vi "3D Experiment Final wii.vi"() -> ()   [LabVIEW 2011]
uses:
  <vilib>/Utility/miscctls.llb/LV3DPointTypeDef.ctl
  <vilib>/Platform/TimedLoop/XDataNode/timing_clust.ctl
  <vilib>/Platform/TimedLoop/XDataNode/nitl_modes.ctl
  <vilib>/Platform/TimedLoop/XDataNode/wakeup.ctl
  <vilib>/Utility/miscctls.llb/LVRGBAColorTypeDef.ctl
  <vilib>/Utility/cursorutil.llb/Set Cursor (Cursor ID).vi
  libs/experiments 2/Action Engines/AE Access VIs/AE - Bluetooth Initialise.vi
  libs/experiments 2/Action Engines/AE Access VIs/AE - Bluetooth Connect All.vi
  <vilib>/Utility/file.llb/Write To Spreadsheet File (DBL).vi
  <vilib>/Utility/file.llb/Write To Spreadsheet File (I64).vi
  <vilib>/Platform/TimedLoop/XDataNode/XDataNode.xnode
  <vilib>/picture/3D Picture Control/NI_3D Picture Control.lvlib
  User32.dll
  <vilib>/Platform/TimedLoop/XDataNode/XDNodeRunTimeDep.lvlib
panel:
  out "initial time 2":u32
  out "initial time":u32
  in  "stop":bool
  out "3D Picture":refnum<vi>(3d-picture)
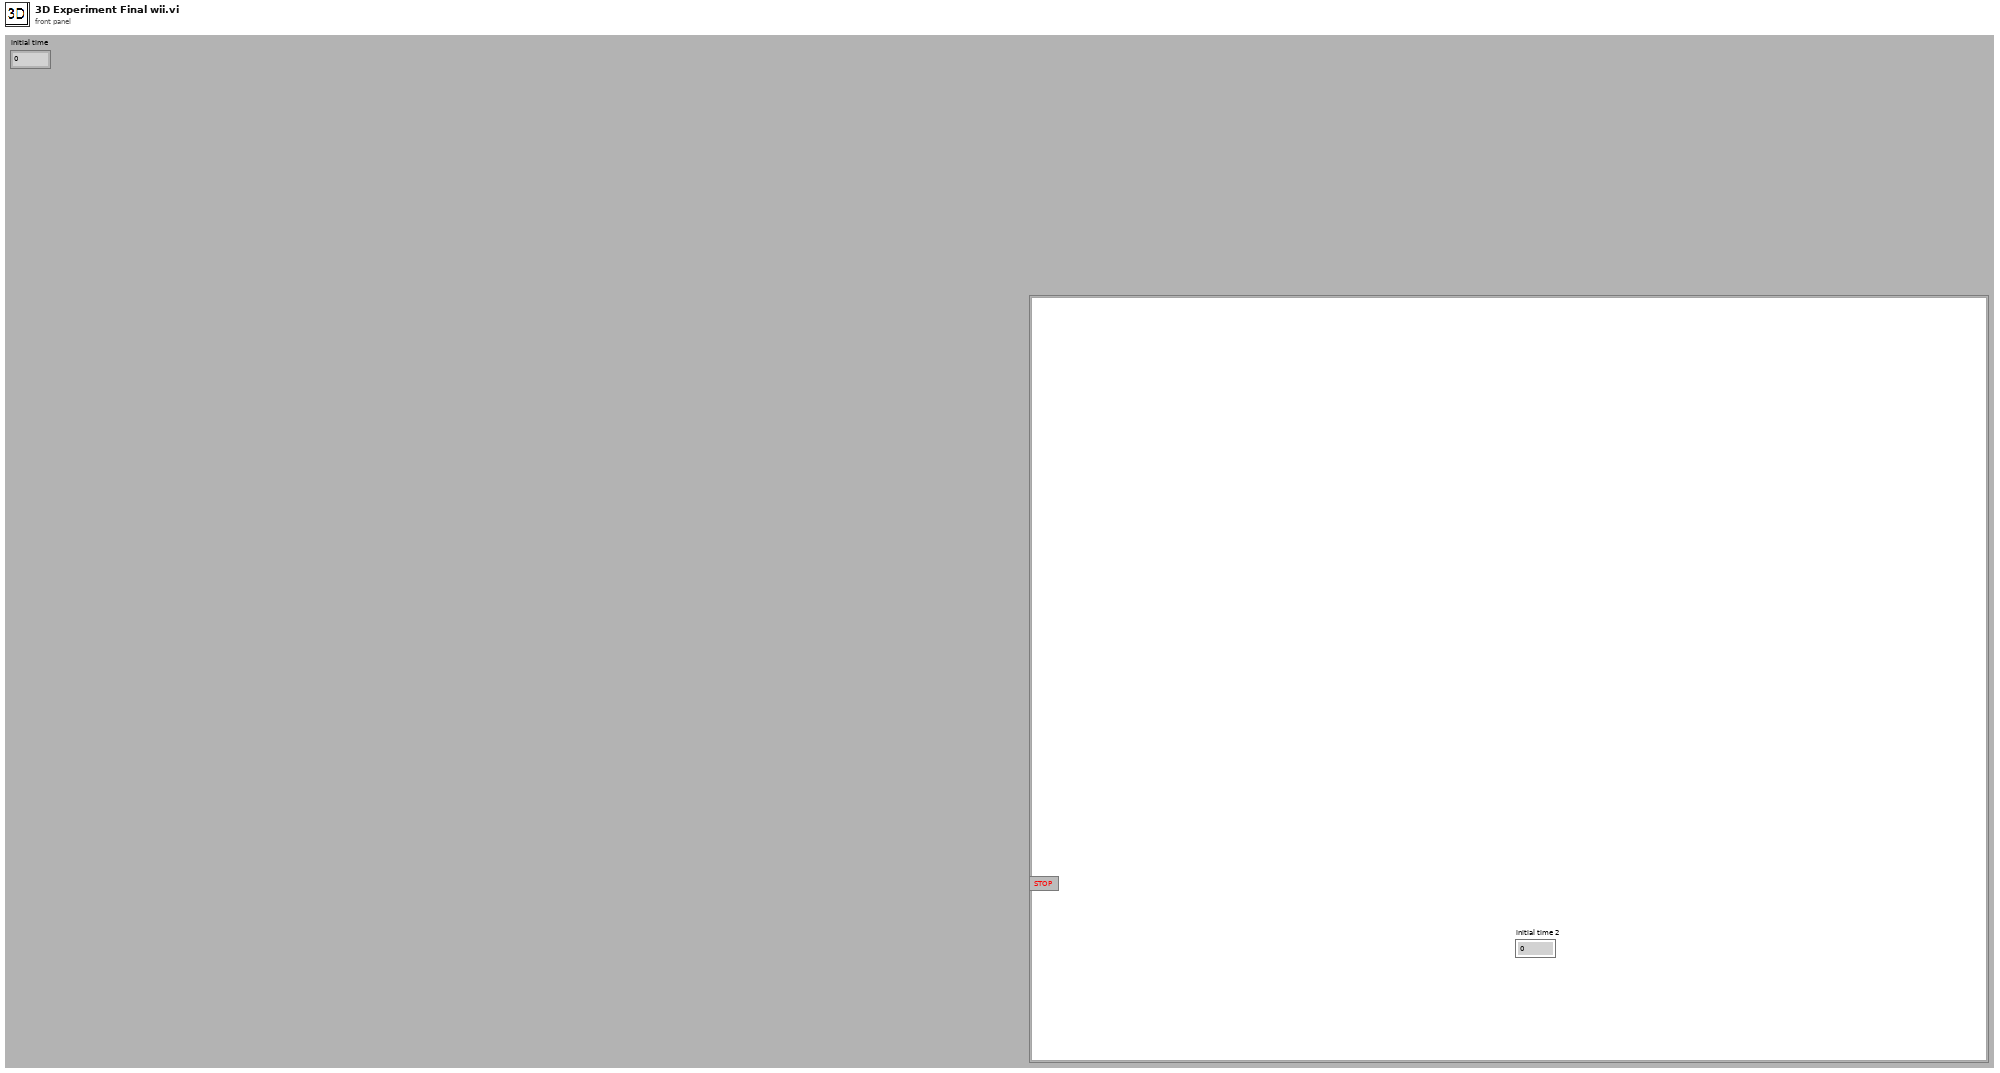
[diagram p1: front panel]
types:
  T1 = enum16{"open", "replace", "create", "open or create", "replace or create", "replace or create with confirmation"}
  T2 = typedef "LV3DPointTypeDef.ctl" = cluster{"X":sgl, "Y":sgl, "Z":sgl}
  T3 = enum16{"Inherit Value", "Points", "Wireframe", "Polygons"}
  T4 = enum16{"Inherit Value", "No Culling", "Cull Back Face", "Cull Front Face", "Cull Both Faces"}
  T5 = enum16{"Zero", "One", "Destination Color", "One Minus Destination Color", "Source Alpha", "One Minus Source Alpha", "Destination Alpha", "One Minus Destination Alpha", "Source Alpha Saturate"}
  T6 = enum16{"Zero", "One", "Source Color", "One Minus Source Color", "Source Alpha", "One Minus Source Alpha", "Destination Alpha", "One Minus Destination Alpha"}
  T7 = enum16{"Normal Bin", "Opaque Bin", "Transparent Bin"}
  T8 = typedef "XDNodeRunTimeDep.lvlib/timing_clust.ctl" = cluster{"Expected End [f-1]":u64, "Actual End [f-1]":u64, "Finished Late? [f-1]":bool, "Expected End [i-1]":u64, "Actual End [i-1]":u64, "Finished Late? [i-1]":bool, "Expected Start [i]":u64, "Actual Start [i]":u64, "Expected Start [f]":u64, "Actual Start [f]":u64, "Source Name":string, "Structure Name":string, "Period":i64, "Deadline":i64, "Offset":i64, "Start":i64, "Priority":i32, "Timeout":i32, "Mode":T9, "Wakeup Reason":T10, "Error":errorcluster, "Source Type":string, "Secondary Source Type":string, "Global End Time":u64, "Global Start Time":u64, "Frame Duration":u64, "Iteration Duration":u64, "Assigned CPU":i32, "I/O Scan Engine Mode":u32}
  T9 = typedef "XDNodeRunTimeDep.lvlib/nitl_modes.ctl" = enum32{"No Change", "Process missed periods, maintain original phase", "Discard missed periods, maintain original phase", "Process missed periods, ignore original phase", "Discard missed periods, ignore original phase"}
  T10 = typedef "XDNodeRunTimeDep.lvlib/wakeup.ctl" = enum32{"Normal", "Aborted", "Asynchronous wakeup", "Timing source error", "Timed loop error", "Timeout"}
  T11 = cluster{"Red":sgl, "Green":sgl, "Blue":sgl, "Alpha":sgl}
  T12 = typedef "LVRGBAColorTypeDef.ctl" = cluster{"Red":sgl, "Green":sgl, "Blue":sgl, "Alpha":sgl}
  T13 = typedef "LVAllMonitorsDisplayTypeDef.ctl" = cluster{"Bounds":cluster{"Left":i16, "Top":i16, "Right":i16, "Bottom":i16}, "Depth":i16}[]
  T14 = cluster{"Bounds":cluster{"Left":i16, "Top":i16, "Right":i16, "Bottom":i16}, "Depth":i16}
  T15 = cluster{"Left":i16, "Top":i16, "Right":i16, "Bottom":i16}
  T16 = cluster{"element":dbl, "Y_scaling":dbl, "element":dbl}
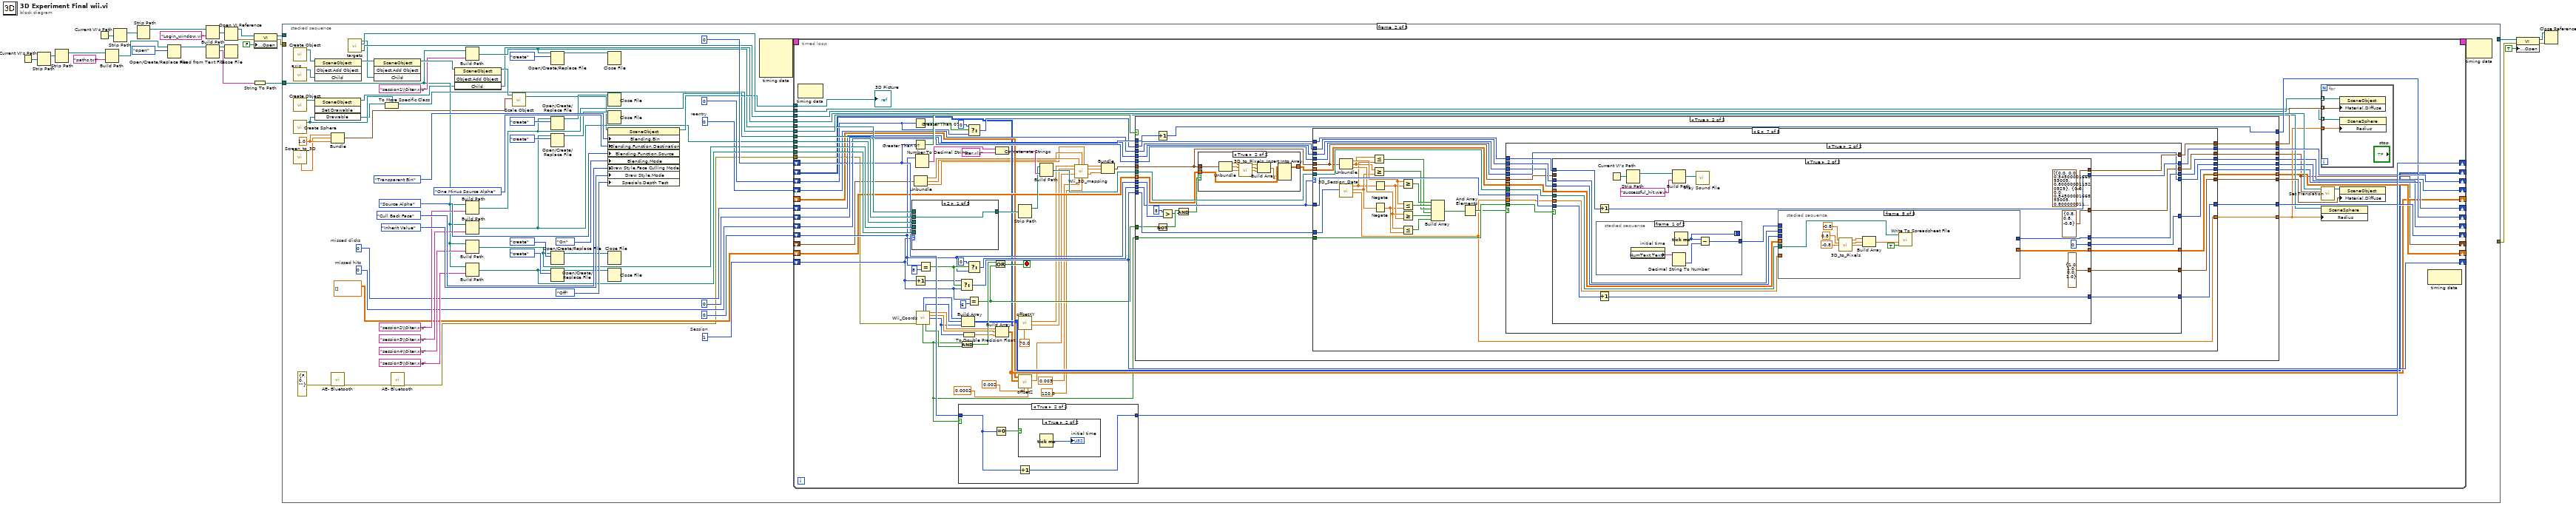
[diagram p0: block diagram]
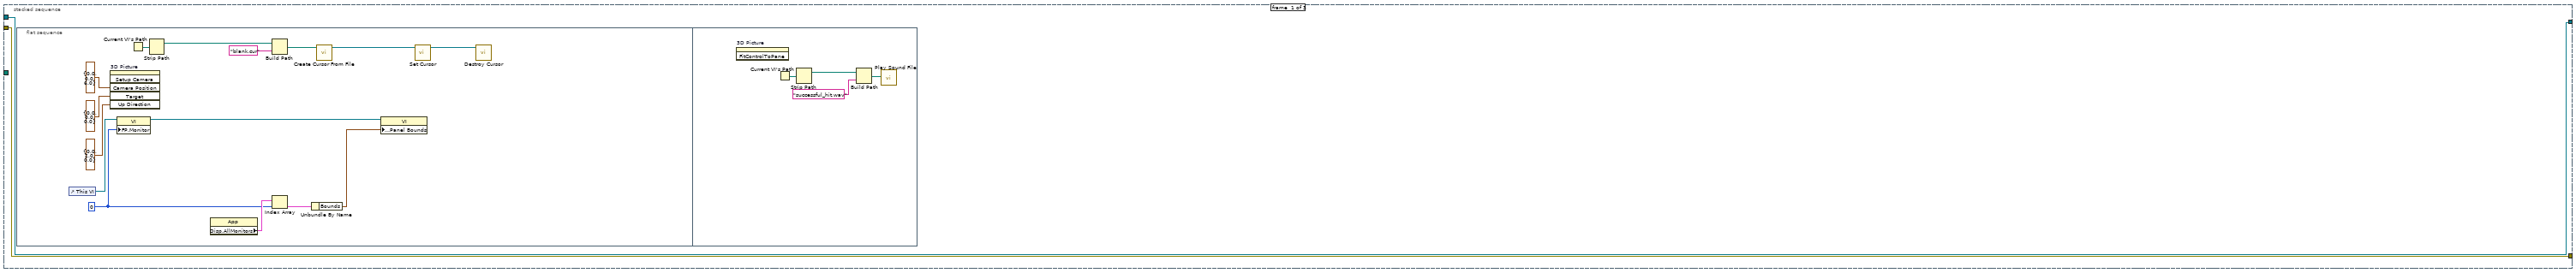
[diagram p2: hidden frame]
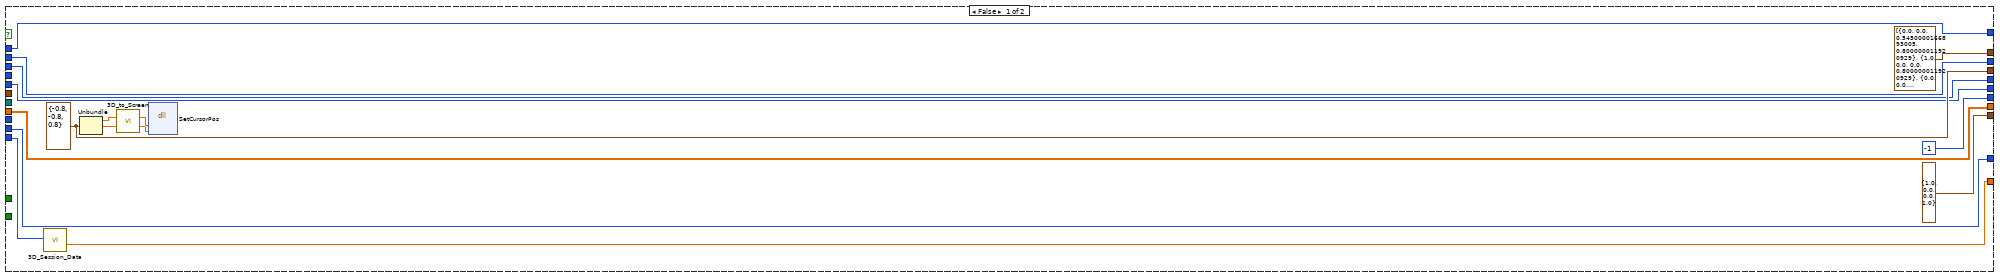
[diagram p7: hidden frame]
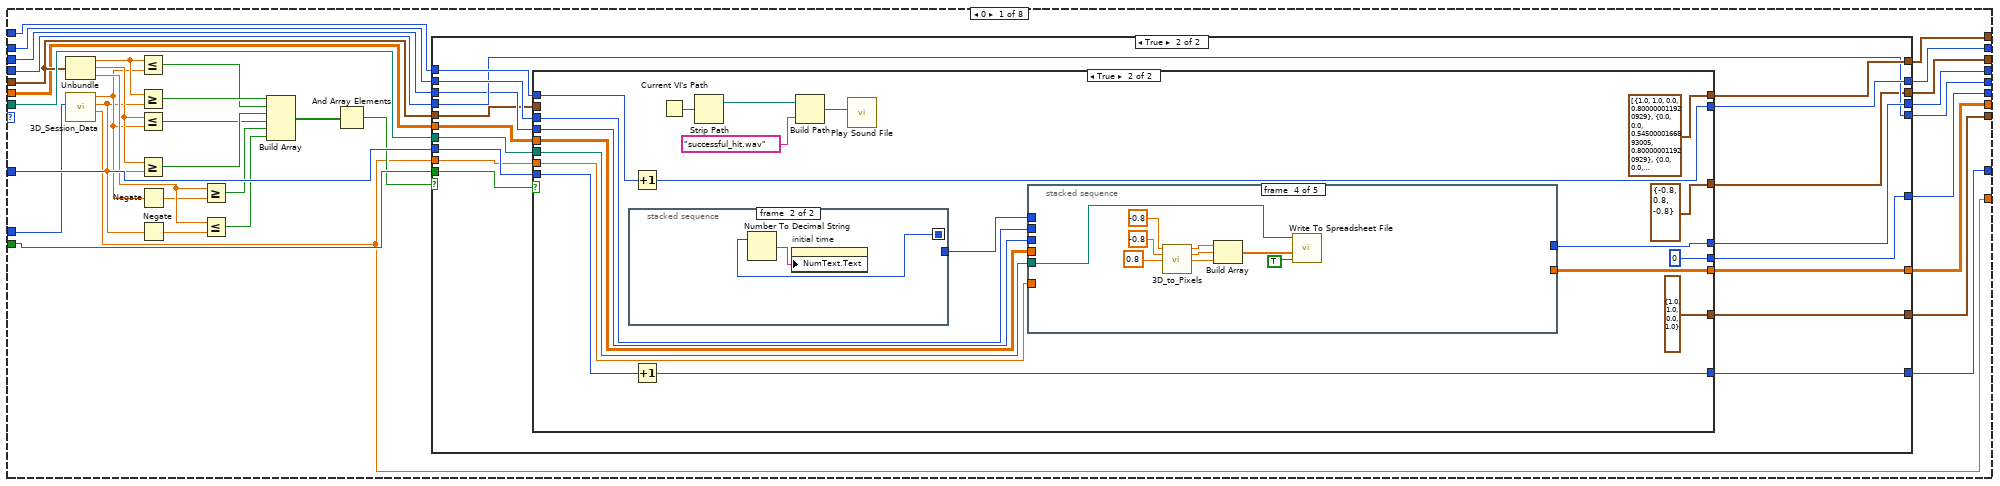
[diagram p9: hidden frame]
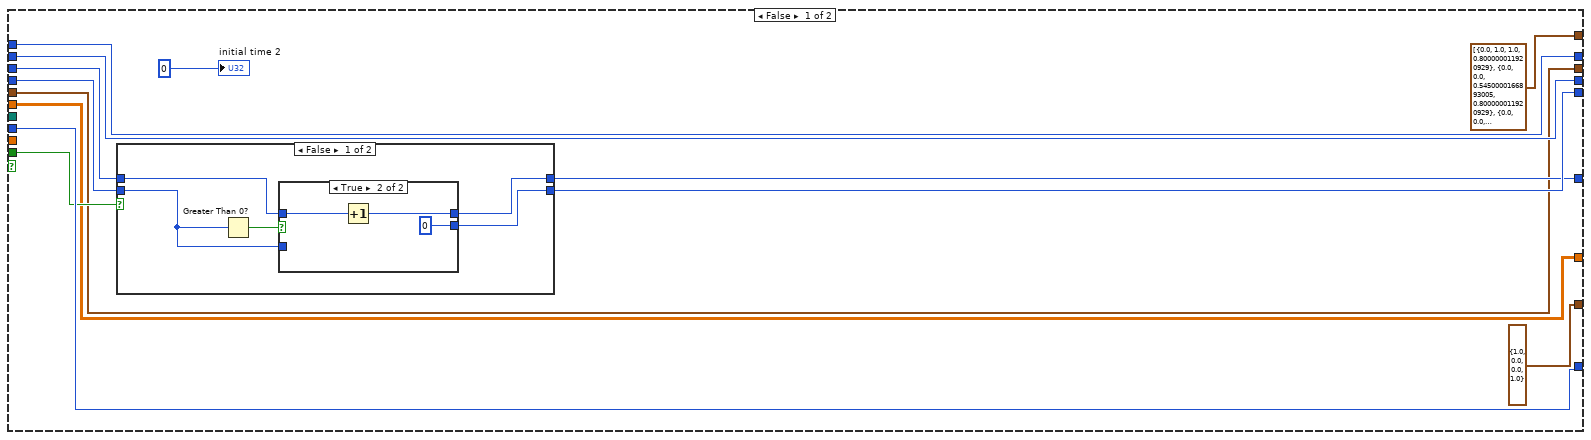
[diagram p10: hidden frame]
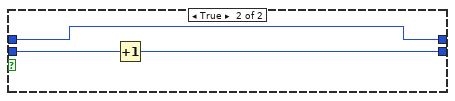
[diagram p12: hidden frame]
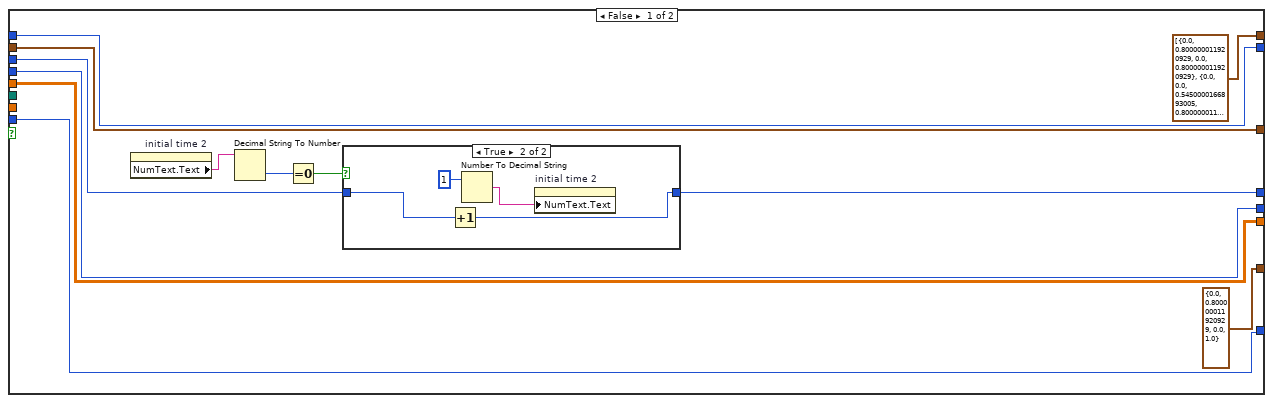
[diagram p13: hidden frame]
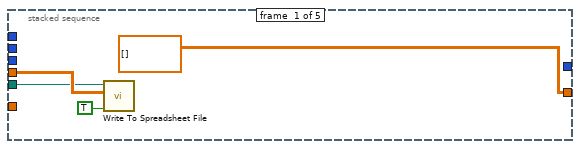
[diagram p15: hidden frame]
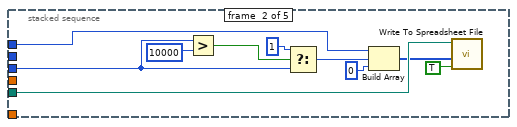
[diagram p16: hidden frame]
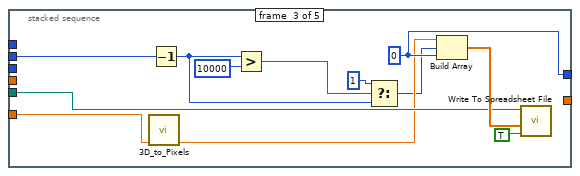
[diagram p17: hidden frame]
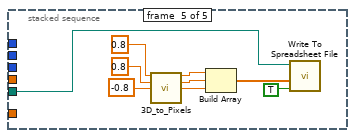
[diagram p18: hidden frame]
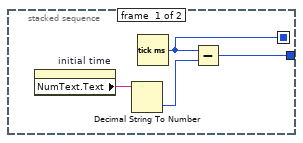
[diagram p19: hidden frame]
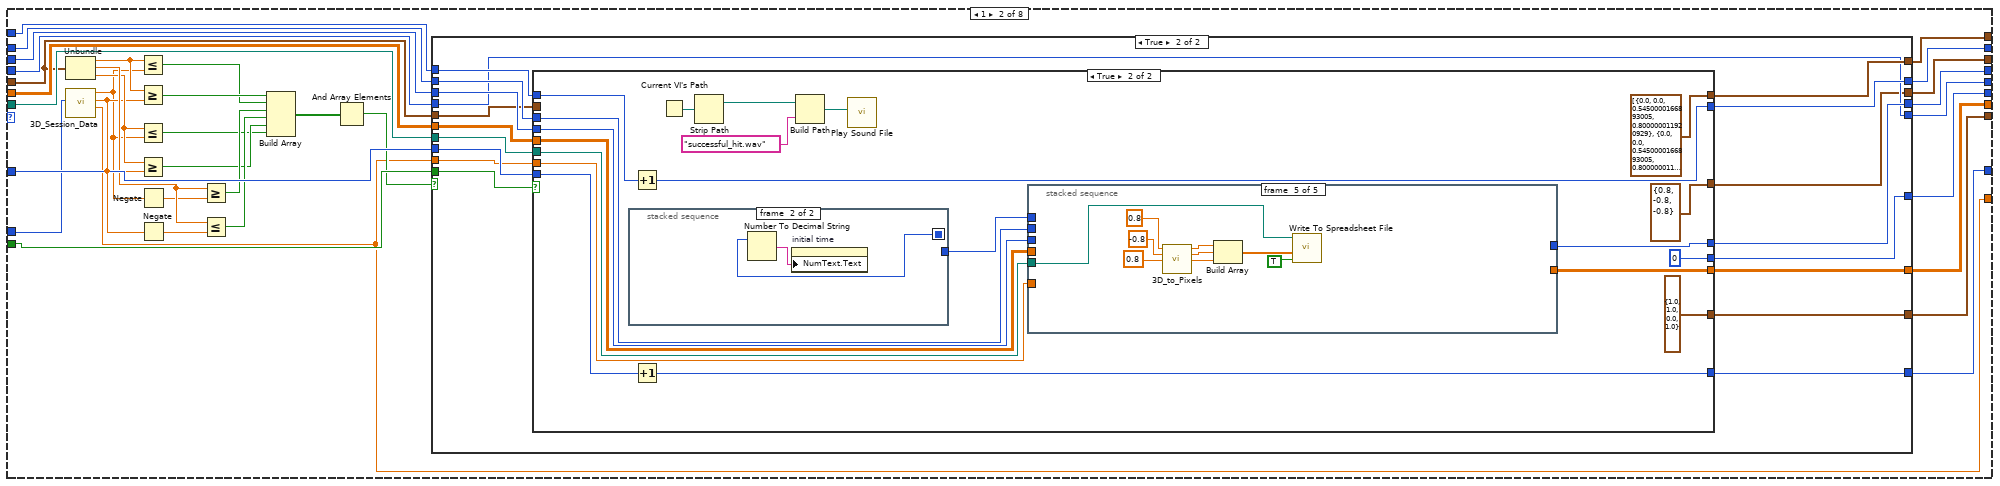
[diagram p20: hidden frame]
diagram:
  n1 = Current VI's Path() -> (path=w1:path)
  n2 = Strip Path(path=w1) -> (stripped path=w2:path)  [unwired: 1 out]
  n3 = Strip Path(path=w2) -> (stripped path=w19:path)  [unwired: 1 out]
  n4 = Current VI's Path() -> (path=w14:path)
  n5 = Build Path(base path=w19, name or relative path="paths.txt") -> (appended path=w22:path)
  n6 = Strip Path(path=w14) -> (stripped path=w11:path)  [unwired: 1 out]
  n7 = Strip Path(path=w11) -> (stripped path=w10:path)  [unwired: 1 out]
  n8 = Open/Create/Replace File(file path (use dialog)=w22, operation (0:open)=T1."open") -> (refnum out=w24:refnum<file>)  [unwired: 4 in, 2 out]
  n9 = Build Path(base path=w10, name or relative path="Login_window.vi") -> (appended path=w12:path)
  n10 = Read from Text File(file (use dialog)=w24) -> (refnum out=w25:refnum<file>, text=w23:string)  [unwired: 3 in, 2 out]
  n11 = Open VI Reference(vi path=w12) -> (vi reference=w17:refnum<vi>, error out=w16:errorcluster)  [unwired: 5 in]
  n12 = Close File(refnum=w25) -> ()  [unwired: 1 in, 2 out]
  n13 = String To Path(string=w23) -> (path=w18:path)
  n14 = property class="VI"(reference=w17, error in=w16, "Front Panel Window:Open"=FALSE) -> (reference out=w9:refnum<vi>, error out=w8:errorcluster)
  n15 = stacked-sequence {
    tunnel: w18 -> [_ w67 _]
    tunnel: w9 -> [w27 _ _]
    tunnel: w8 -> [w26 _ _]
    tunnel: [w27 _ _] -> w4
    tunnel: [w26 _ _] -> w3
    frame #0 {
      n16 = flat-sequence {
        frame #0 {
          w39 = u16 0 ("Front Panel Window:Monitor")
          n17 = control-ref of="This VI"() -> (w37:refnum<vi>)
          n18 = invoke on="3D Picture" class="SceneGraphDisp (strict)" method="Setup Camera"("Camera Position"=T2 {"X"=0.0, "Y"=0.0, "Z"=6.0}, "Target"=T2 {"X"=0.0, "Y"=0.0, "Z"=0.0}, "Up Direction"=T2 {"X"=0.0, "Y"=2.0, "Z"=0.0}) -> ()  [unwired: 3 in, 6 out]
          n19 = property class="VI"(reference=w37, "FP.Monitor"=w39) -> (reference out=w41:refnum<vi>)  [unwired: 1 in, 1 out]
          n20 = Current VI's Path() -> (path=w36:path)
          n21 = Strip Path(path=w36) -> (stripped path=w35:path)  [unwired: 1 out]
          n22 = property class="App"() -> ("Disp.AllMonitors"=w40:T13)  [unwired: 2 in, 2 out]
          n23 = Build Path(base path=w35, name or relative path="blank.cur") -> (appended path=w33:path)
          n24 = Index Array(array=w40, index=w39) -> (element=w38:T14)
          n25 = Unbundle By Name(w38) -> ("Bounds"=w42:T15)
          n26 = call <vilib>:"Create Cursor From File.vi"("cursor file"=w33) -> ("cursor ID"=w32:refnum<k1>)  [unwired: 9 in, 1 out]
          n27 = property class="VI"(reference=w41, "Front Panel Window:Panel Bounds"=w42) -> ()  [unwired: 1 in, 2 out]
          n28 = call-poly <vilib>:"Set Cursor.vi"("cursor ID"=w32) -> ("previous cursor ID"=w31:refnum<k1>)  [unwired: 9 in, 1 out]
          n29 = call <vilib>:"Destroy Cursor.vi"("cursor ID"=w31) -> ()  [unwired: 9 in, 1 out]
        }
        frame #1 {
          n30 = invoke on="3D Picture" class="SceneGraphDisp (strict)" method="FitControlToPane"() -> ()  [unwired: 3 in, 3 out]
          n31 = Current VI's Path() -> (path=w45:path)
          n32 = Strip Path(path=w45) -> (stripped path=w44:path)  [unwired: 1 out]
          n33 = Build Path(base path=w44, name or relative path="successful_hit.wav") -> (appended path=w46:path)
          n34 = call <vilib>:"Play Sound File.vi"("path"=w46) -> ()  [unwired: 9 in, 2 out]
        }
      }
    }
    frame #1 {
      w54 = 1.0 ("element")
      w55 = 0  # missed clicks
      w56 = 0  # missed hits
      w57 = 0  # reentry
      w96 = 1  # Session
      n35 = call <vilib>:"Create Object.vi"() -> ("Scene:New Object"=w100:refnum<vi>)  [unwired: 10 in, 1 out]
      n36 = call "axis.vi"() -> ("reference out"=w59:refnum<vi>)  [unwired: 11 in]
      n37 = call <vilib>:"Create Object.vi"() -> ("Scene:New Object"=w101:refnum<vi>)  [unwired: 10 in, 1 out]
      n38 = call <vilib>:"Create Sphere.vi"() -> ("New Sphere Refnum"=w94:refnum<vi>)  [unwired: 10 in, 1 out]
      n39 = call "Screen_to_3D.vi"() -> ("Y_scaling"=w51:dbl)  [unwired: 13 in, 6 out]
      n40 = invoke class="SceneObject" method="Object.Add Object"(reference=w100, "Child"=w59) -> (reference out=w99:refnum<vi>)  [unwired: 2 in, 3 out]
      n41 = invoke class="SceneObject" method="Set Drawable"(reference=w101, "Drawable"=w94) -> (reference out=w60:refnum<vi>, "Drawable"=w93:refnum<vi>)  [unwired: 2 in, 2 out]
      n42 = call-poly "AE- Bluetooth.vi"("error in (no error)"=errorcluster {"status"=FALSE, "code"=0, "source"=""}) -> ("error out"=w48:errorcluster)  [unwired: 10 in]
      n43 = Bundle("element"=w54, "Y_scaling"=w51, "element"=w54) -> (w53:T16)  [unwired: 1 in]
      n44 = call "targets.vi"() -> ("objects"=w95:refnum<vi>[], "shperes"=w91:refnum<vi>[], "Scene:New Object"=w58:refnum<vi>)  [unwired: 8 in]
      n45 = invoke class="SceneObject" method="Object.Add Object"(reference=w99, "Child"=w58) -> (reference out=w98:refnum<vi>)  [unwired: 2 in, 3 out]
      n46 = To More Specific Class(target class=w94, reference=w93) -> (specific class reference=w92:refnum<vi>)  [unwired: 1 in, 1 out]
      n47 = call-poly "AE- Bluetooth.vi"("error in (no error)"=w48) -> ("error out"=w47:errorcluster)  [unwired: 9 in, 1 out]
      n48 = invoke class="SceneObject" method="Object.Add Object"(reference=w98, "Child"=w60) -> (reference out=w97:refnum<vi>, "Child"=w61:refnum<vi>)  [unwired: 2 in, 2 out]
      n49 = Build Path(base path=w67, name or relative path="session1\\0iter.xls") -> (appended path=w62:path)
      n50 = Build Path(base path=w67, name or relative path="session2\\0iter.xls") -> (appended path=w63:path)
      n51 = Build Path(base path=w67, name or relative path="session3\\0iter.xls") -> (appended path=w65:path)
      n52 = Build Path(base path=w67, name or relative path="session4\\0iter.xls") -> (appended path=w64:path)
      n53 = Build Path(base path=w67, name or relative path="session5\\0iter.xls") -> (appended path=w66:path)
      n54 = call <vilib>:"Scale Object.vi"("Scale"=w53, "Scene.Object In"=w97) -> ("Scene.Object Out"=w52:refnum<vi>)  [unwired: 8 in, 1 out]
      n55 = Open/Create/Replace File(file path (use dialog)=w62, operation (0:open)=T1."create") -> (refnum out=w75:refnum<file>)  [unwired: 4 in, 2 out]
      n56 = Open/Create/Replace File(file path (use dialog)=w63, operation (0:open)=T1."create") -> (refnum out=w77:refnum<file>)  [unwired: 4 in, 2 out]
      n57 = Open/Create/Replace File(file path (use dialog)=w65, operation (0:open)=T1."create") -> (refnum out=w72:refnum<file>)  [unwired: 4 in, 2 out]
      n58 = Open/Create/Replace File(file path (use dialog)=w64, operation (0:open)=T1."create") -> (refnum out=w69:refnum<file>)  [unwired: 4 in, 2 out]
      n59 = Open/Create/Replace File(file path (use dialog)=w66, operation (0:open)=T1."create") -> (refnum out=w70:refnum<file>)  [unwired: 4 in, 2 out]
      n60 = Close File(refnum=w75) -> ()  [unwired: 1 in, 2 out]
      n61 = Close File(refnum=w77) -> ()  [unwired: 1 in, 2 out]
      n62 = Close File(refnum=w72) -> ()  [unwired: 1 in, 2 out]
      n63 = property class="SceneObject"(reference=w52, "Blending.Bin"=T7."Transparent Bin" ("Blending:Bin"), "Blending.Function.Destination"=T6."One Minus Source Alpha" ("Blending:Function:Destination"), "Blending.Function.Source"=T5."Source Alpha" ("Blending:Function:Source"), "Blending.Mode"=enum16{"Inherit Value", "Off", "On"}."On" ("Blending:Mode"), "Draw Style.Face Culling Mode"=T4."Cull Back Face" ("Draw Style:Face Culling Mode"), "Draw Style.Mode"=T3."Inherit Value" ("Draw Style:Mode"), "Specials.Depth Test"=enum16{"Inherit Value", "Off", "On"}."Off" ("Specials:Depth Test")) -> (reference out=w83:refnum<vi>)  [unwired: 1 in, 1 out]
      n64 = Close File(refnum=w69) -> ()  [unwired: 1 in, 2 out]
      n65 = Close File(refnum=w70) -> ()  [unwired: 1 in, 2 out]
      n66 = node-c288() -> (w107:T8)  [unwired: 4 in]
      n67 = timed-loop {
        shift-right: [w188] -> _
        shift-left: 0 ("y") -> [w152]
        shift-right: [w186] -> _
        shift-left: 0 ("y") -> [w142]
        shift-right: [w122] -> _
        shift-left: _ -> [w121]
        shift-right: [w185] -> _
        shift-left: 0 ("y") -> [w147]
        timing: w107 -> [_]
        timing-out: [_] -> w106
        shift-right: [w141] -> _
        shift-left: w96 -> [w140]
        shift-right: [w181] -> _
        shift-left: 0 ("y") -> [w182]
        tunnel: w83 -> [w180]
        tunnel: w61 -> [w179]
        tunnel: w95 -> [w176]
        tunnel: w92 -> [w174]
        tunnel: w91 -> [w172]
        tunnel: w66 -> [w168]
        tunnel: w65 -> [w167]
        tunnel: w64 -> [w166]
        tunnel: w63 -> [w165]
        tunnel: w62 -> [w164]
        shift-right: [w159] -> _
        shift-left: w57 -> [w160]
        shift-right: [w153] -> _
        shift-left: w56 -> [w156]
        shift-right: [w154] -> _
        shift-left: w55 -> [w155]
        shift-right: [w137] -> _
        shift-left: dbl[][] [] -> [w138]
        tunnel: w47 -> [w131]
        shift-right: [w130] -> _
        shift-left: _ -> [w129]
        shift-right: [w128] -> _
        shift-left: _ -> [w127]
        stop <- w157 stop-if-true
        n68 = node-c288() -> ()  [unwired: 1 in, 1 out]
        n69 = case shown="2" w140 {
          tunnel: w168 -> [_ _ _ w192 _]
          tunnel: w166 -> [_ _ w191 _ _]
          tunnel: w167 -> [_ w190 _ _ _]
          tunnel: w165 -> [w189 _ _ _ _]
          tunnel: w164 -> [_ _ _ _ w193]
          tunnel: [w189 w190 w191 w192 w193] -> w161
          frame 2 {
          }
          frame 3 {
          }
          frame 4 {
          }
          frame 5 {
          }
          frame 1, Default {
          }
        }
        n70 = Greater Than 0?(x=w147) -> (x > 0?=w150:bool)
        n71 = Greater Than 0?(x=w152) -> (x > 0?=w187:bool)
        n72 = Increment(x=w140) -> (x+1=w143:i32)
        n73 = Unbundle(w121) -> ("X_3D"=w120:dbl, "Y_3D"=w119:dbl, "y"=w118:dbl)
        n74 = Number To Decimal String(number=w142) -> (decimal integer string=w169:string)  [unwired: 1 in]
        n75 = call "Wii_Coords.vi"("error in (no error)"=w131) -> ("Raw X Values"=w134:i32[], "Raw Y Values"=w133:i32[], "X Values"=w136:sgl[], "Y Values"=w135:sgl[], "Sizes"=w132:i32[], "B"=w112:bool, "Home"=w125:bool)  [unwired: 7 in, 1 out]
        n76 = Equal?(x=w142, y=8) -> (x = y?=w146:bool)
        n77 = case shown="True" w112 {
          tunnel: w152 -> [w1589 w1590]
          tunnel: [w1589 w1592] -> w188
          frame False {
          }
          frame True {
            n78 = Equal To 0?(x=w1590) -> (x = 0?=w1591:bool)
            n79 = Increment(x=w1590) -> (x+1=w1592:i32)
            n80 = case shown="True" w1591 {
              frame False {
              }
              frame True {
                n81 = Tick Count (ms)() -> (millisecond timer value=→"initial time":u32)
              }
            }
          }
        }
        n82 = Select(t=w143, s=w146, f=w140) -> (s? t:f=w141:i32)
        n83 = And(x=w112, y=w125) -> (x .and. y?=w158:bool)
        n84 = Build Array(w134, w133, w132) -> (w128:i32[][])
        n85 = To Double Precision Float(number=w132) -> (double precision float=w126:dbl[])
        n86 = Select(t=0 ("y"), s=w150, f=w147) -> (s? t:f=w148:i32)
        n87 = Select(t=0 ("y"), s=w146, f=w142) -> (s? t:f=w144:i32)
        n88 = Equal?(x=w140, y=6) -> (x = y?=w139:bool)
        n89 = Or(x=w158, y=w139) -> (x .or. y?=w157:bool)
        n90 = Concatenate Strings(w169, "iter.xls" ("name or relative path")) -> (w170:string)
        n91 = Build Array(w136, w135, w126) -> (w130:dbl[][])
        n92 = Strip Path(path=w161) -> (stripped path=w162:path)  [unwired: 1 out]
        n93 = call "offsetXY.vi"("Thres"=70.0, "Previous"=w127, "Current"=w128) -> ("OffsetY"=w124:dbl, "OffsetX"=w123:dbl)  [unwired: 7 in]
        n94 = call "offsetZ.vi"("Low Thres"=0.0002, "Up Thres"=0.002 ("Thres"), "Current"=w130, "Previous"=w129) -> ("OffsetZ"=w113:dbl)  [unwired: 7 in]
        n95 = Build Path(base path=w162, name or relative path=w170) -> (appended path=w163:path)
        n96 = call "Wii_3D_mapping.vi"("Wii_X_off"=w123, "previous_X_3D"=w120, "previous_Y_3D"=w119, "previous_Z_3D"=w118, "Wii_Y_off"=w124, "Wii_Z_off"=w113, "X_Y_speed"=0.003, "Z_speed"=120.0) -> ("X_3D"=w109:dbl, "Y_3D"=w108:dbl, "Z_3D"=w110:dbl)  [unwired: 5 in]
        n97 = Bundle("X_3D"=w109, "Y_3D"=w108, "Z_3D"=w110) -> (w151:cluster{"X_3D":dbl, "Y_3D":dbl, "Z_3D":dbl})  [unwired: 1 in]
        n98 = case shown="True" w187 {
          tunnel: w151 -> [_ w225]
          tunnel: [w212 w226] -> w122
          tunnel: [T12[] [{"Red"=0.0, "Green"=0.0, "Blue"=0.545, "Alpha"=0.8}, {"Red"=1.0, "Green"=0.0, "Blue"=0.0, "Alpha"=0.8}, {"Red"=0.0, "Green"=0.0, "Blue"=0.545, "Alpha"=0.8}, {"Red"=0.0, "Green"=0.0, "Blue"=0.545, "Alpha"=0.8}, {"Red"=0.0, "Green"=0.0, "Blue"=0.545, "Alpha"=0.8}, {"Red"=0.0, "Green"=0.0, "Blue"=0.545, "Alpha"=0.8}, {"Red"=0.0, "Green"=0.0, "Blue"=0.545, "Alpha"=0.8}, {"Red"=0.0, "Green"=0.0, "Blue"=0.545, "Alpha"=0.8}] ("Array") w244] -> w175
          tunnel: w144 -> [w213 w223]
          tunnel: w112 -> [_ w242]
          tunnel: [T11 {"Red"=1.0, "Green"=0.0, "Blue"=0.0, "Alpha"=1.0} ("Color") w243] -> w178
          tunnel: [w213 w241] -> w186
          tunnel: w148 -> [w211 w240]
          tunnel: [w211 w239] -> w185
          tunnel: w141 -> [w209 w238]
          tunnel: w182 -> [w210 w237]
          tunnel: [w210 w236] -> w181
          tunnel: [w208 w235] -> w173
          tunnel: w163 -> [_ w231]
          tunnel: w160 -> [w207 w234]
          tunnel: [w207 w233] -> w159
          tunnel: w142 -> [_ w232]
          tunnel: w156 -> [w206 w230]
          tunnel: w155 -> [_ w229]
          tunnel: [-1 ("y") w228] -> w154
          tunnel: [w206 w227] -> w153
          tunnel: w139 -> [_ w222]
          tunnel: w138 -> [w200 w218]
          tunnel: [w200 w216] -> w137
          frame False {
            w212 = cluster{dbl, dbl, "y":dbl} {-0.8, -0.8, "y"=0.8}
            n99 = call "3D_Session_Data.vi"("Session"=w209) -> ("Radius"=w208:sgl)  [unwired: 8 in, 2 out]
            n100 = Unbundle(w212) -> (w205:dbl, w204:dbl)  [unwired: 1 out]
            n101 = call "3D_to_Screen.vi"("X_3D"=w205, "Y_3D"=w204) -> ("X"=w203:dbl, "Y"=w202:dbl)  [unwired: 11 in, 1 out]
            n102 = dll-call lib="User32.dll" fn="SetCursorPos"(w203, w202) -> ()  [unwired: 6 in, 2 out]
          }
          frame True {
            n103 = Increment(x=w237) -> (x+1=w236:i32)
            n104 = Not(x=w222) -> (.not. x?=w221:bool)
            n105 = Greater?(x=8 ("y"), y=w232) -> (0:w220:bool)
            n106 = And(x=w221, y=w220) -> (x .and. y?=w219:bool)
            n107 = case shown="True" w219 {
              tunnel: w225 -> [_ w255]
              tunnel: w218 -> [w245 w248]
              tunnel: [w245 w246] -> w217
              frame False {
              }
              frame True {
                n108 = Unbundle(w255) -> ("X_3D"=w254:dbl, "Y_3D"=w253:dbl, "Z_3D"=w252:dbl)
                n109 = call "3D_to_Pixels.vi"("X_3D"=w254, "Y_3D"=w253, "Z_3D"=w252) -> ("X_pixels"=w251:dbl, "Y_pixels"=w250:dbl, "Z_pixels"=w249:dbl)  [unwired: 9 in, 1 out]
                n110 = Build Array(w251, w250, w249) -> (w247:dbl[])
                n111 = Insert Into Array(array=w248, new element=w247) -> (w246:dbl[][])  [unwired: 2 in]
              }
            }
            n112 = case shown="6" w223 {
              tunnel: [w290 w456 w623 w790 w955 w1122 w1289 w1456] -> w244
              tunnel: w225 -> [w259 w424 w591 w758 w924 w1090 w1256 w1424]
              tunnel: [w289 w455 w622 w789 w954 w1121 w1288 w1455] -> w243
              tunnel: w242 -> [w288 w443 w621 w788 w953 w1120 w1287 w1454]
              tunnel: w223 -> [w287 w454 w620 w787 w952 w1119 w1286 w1453]
              tunnel: [w286 w453 w619 w786 w951 w1118 w1285 w1452] -> w241
              tunnel: w240 -> [w274 w452 w618 w785 w950 w1117 w1284 w1451]
              tunnel: [w273 w451 w617 w784 w949 w1116 w1283 w1450] -> w239
              tunnel: w238 -> [w272 w423 w590 w756 w925 w1089 w1257 w1423]
              tunnel: [w266 w422 w589 w759 w923 w1088 w1255 w1422] -> w235
              tunnel: w231 -> [w267 w450 w616 w783 w948 w1115 w1282 w1449]
              tunnel: w234 -> [w264 w448 w614 w781 w946 w1113 w1280 w1448]
              tunnel: [w265 w449 w615 w782 w947 w1114 w1281 w1447] -> w233
              tunnel: w230 -> [w263 w447 w613 w780 w945 w1112 w1279 w1446]
              tunnel: w229 -> [w262 w446 w612 w779 w944 w1111 w1278 w1445]
              tunnel: [w260 w444 w610 w777 w942 w1109 w1276 w1444] -> w228
              tunnel: [w261 w445 w611 w778 w943 w1110 w1277 w1443] -> w227
              tunnel: [w258 w442 w609 w776 w941 w1108 w1275 w1442] -> w226
              tunnel: w217 -> [w257 w440 w608 w775 w940 w1107 w1274 w1441]
              tunnel: [w256 w441 w607 w774 w939 w1106 w1273 w1440] -> w216
              frame 0 {
                n113 = Unbundle(w259) -> ("X_3D"=w285:dbl, "Y_3D"=w284:dbl, "Z_3D"=w283:dbl)
                n114 = call "3D_Session_Data.vi"("Session"=w272) -> ("Radius"=w266:sgl, "min"=w270:dbl, "max"=w271:dbl)  [unwired: 8 in]
                n115 = Less Or Equal?(x=w285, y=w271) -> (x <= y?=w281:bool)
                n116 = Greater Or Equal?(x=w285, y=w270) -> (x >= y?=w282:bool)
                n117 = Less Or Equal?(x=w284, y=w271) -> (x <= y?=w279:bool)
                n118 = Greater Or Equal?(x=w284, y=w270) -> (x >= y?=w280:bool)
                n119 = Negate(x=w271) -> (-x=w269:dbl)
                n120 = Negate(x=w270) -> (-x=w268:dbl)
                n121 = Greater Or Equal?(x=w283, y=w269) -> (x >= y?=w278:bool)
                n122 = Less Or Equal?(x=w283, y=w268) -> (x <= y?=w277:bool)
                n123 = Build Array(w282, w281, w280, w279, w278, w277) -> (w276:bool[])
                n124 = And Array Elements(Boolean array=w276) -> (logical AND=w275:bool)
                n125 = case shown="True" w275 {
                  tunnel: [T12[] [{"Red"=0.0, "Green"=1.0, "Blue"=1.0, "Alpha"=0.8}, {"Red"=0.0, "Green"=0.0, "Blue"=0.545, "Alpha"=0.8}, {"Red"=0.0, "Green"=0.0, "Blue"=0.545, "Alpha"=0.8}, {"Red"=0.0, "Green"=0.0, "Blue"=0.545, "Alpha"=0.8}, {"Red"=0.0, "Green"=0.0, "Blue"=0.545, "Alpha"=0.8}, {"Red"=0.0, "Green"=0.0, "Blue"=0.545, "Alpha"=0.8}, {"Red"=0.0, "Green"=0.0, "Blue"=0.545, "Alpha"=0.8}, {"Red"=0.0, "Green"=0.0, "Blue"=0.545, "Alpha"=0.8}] ("Array") w334] -> w290
                  tunnel: [T11 {"Red"=1.0, "Green"=0.0, "Blue"=0.0, "Alpha"=1.0} ("Color") w333] -> w289
                  tunnel: w288 -> [w293 w332]
                  tunnel: w287 -> [w301 w331]
                  tunnel: [w301 w330] -> w286
                  tunnel: w274 -> [w300 w329]
                  tunnel: [w300 w328] -> w273
                  tunnel: w267 -> [_ w327]
                  tunnel: w266 -> [_ w326]
                  tunnel: [w299 w325] -> w265
                  tunnel: w264 -> [w299 w324]
                  tunnel: w263 -> [w297 w323]
                  tunnel: w262 -> [w296 w322]
                  tunnel: [w295 w323] -> w261
                  tunnel: [w294 w321] -> w260
                  tunnel: w259 -> [w292 w320]
                  tunnel: [w292 w319] -> w258
                  tunnel: w257 -> [w291 w318]
                  tunnel: [w291 w317] -> w256
                  frame False {
                    n126 = case shown="False" w293 {
                      tunnel: w297 -> [w304 w316]
                      tunnel: [w305 w315] -> w295
                      tunnel: w296 -> [w307 w314]
                      tunnel: [w306 w314] -> w294
                      frame False {
                        n127 = Greater Than 0?(x=w304) -> (x > 0?=w308:bool)
                        n128 = case shown="True" w308 {
                          tunnel: w307 -> [w310 w313]
                          tunnel: [w310 w312] -> w306
                          tunnel: w304 -> [w309 _]
                          tunnel: [w309 0 ("y")] -> w305
                          frame False {
                          }
                          frame True {
                            n129 = Increment(x=w313) -> (x+1=w312:i32)
                          }
                        }
                      }
                      frame True {
                        n130 = Increment(x=w316) -> (x+1=w315:i32)
                      }
                    }
                    "initial time 2" <- u32 0 ("initial time 2")
                  }
                  frame True {
                    n131 = case shown="True" w332 {
                      tunnel: [T12[] [{"Red"=0.0, "Green"=0.8, "Blue"=0.0, "Alpha"=0.8}, {"Red"=0.0, "Green"=0.0, "Blue"=0.545, "Alpha"=0.8}, {"Red"=0.0, "Green"=0.0, "Blue"=0.545, "Alpha"=0.8}, {"Red"=0.0, "Green"=0.0, "Blue"=0.545, "Alpha"=0.8}, {"Red"=0.0, "Green"=0.0, "Blue"=0.545, "Alpha"=0.8}, {"Red"=0.0, "Green"=0.0, "Blue"=0.545, "Alpha"=0.8}, {"Red"=0.0, "Green"=0.0, "Blue"=0.545, "Alpha"=0.8}, {"Red"=0.0, "Green"=0.0, "Blue"=0.545, "Alpha"=0.8}] ("Array") T12[] [{"Red"=1.0, "Green"=1.0, "Blue"=0.0, "Alpha"=0.8}, {"Red"=0.0, "Green"=0.0, "Blue"=0.545, "Alpha"=0.8}, {"Red"=0.0, "Green"=0.0, "Blue"=0.545, "Alpha"=0.8}, {"Red"=0.0, "Green"=0.0, "Blue"=0.545, "Alpha"=0.8}, {"Red"=0.0, "Green"=0.0, "Blue"=0.545, "Alpha"=0.8}, {"Red"=0.0, "Green"=0.0, "Blue"=0.545, "Alpha"=0.8}, {"Red"=0.0, "Green"=0.0, "Blue"=0.545, "Alpha"=0.8}, {"Red"=0.0, "Green"=0.0, "Blue"=0.545, "Alpha"=0.8}] ("Array")] -> w334
                      tunnel: [T11 {"Red"=0.0, "Green"=0.8, "Blue"=0.0, "Alpha"=1.0} ("Color") T11 {"Red"=1.0, "Green"=1.0, "Blue"=0.0, "Alpha"=1.0} ("Color")] -> w333
                      tunnel: w331 -> [w344 w369]
                      tunnel: [w344 w368] -> w330
                      tunnel: w329 -> [w343 w355]
                      tunnel: [w343 w367] -> w328
                      tunnel: w327 -> [_ w361]
                      tunnel: w326 -> [_ w360]
                      tunnel: [w338 w359] -> w325
                      tunnel: w324 -> [w339 w358]
                      tunnel: w322 -> [w337 w357]
                      tunnel: [w337 0 ("x")] -> w321
                      tunnel: w320 -> [w336 _]
                      tunnel: [w336 cluster{dbl, dbl, "y":dbl} {-0.8, 0.8, "y"=-0.8}] -> w319
                      tunnel: w318 -> [w335 w353]
                      tunnel: [w335 w352] -> w317
                      frame False {
                        n132 = property on="initial time 2" class="DigNum (strict)"() -> ("NumText.Text"=w341:string)  [unwired: 2 in, 2 out]
                        n133 = Decimal String To Number(string=w341) -> (number=w340:i32)  [unwired: 2 in, 1 out]
                        n134 = Equal To 0?(x=w340) -> (x = 0?=w342:bool)
                        n135 = case shown="True" w342 {
                          tunnel: w339 -> [w347 w351]
                          tunnel: [w347 w350] -> w338
                          frame False {
                          }
                          frame True {
                            n136 = Increment(x=w351) -> (x+1=w350:u32)
                            n137 = Number To Decimal String(number=1) -> (decimal integer string=w349:string)  [unwired: 1 in]
                            n138 = property on="initial time 2" class="DigNum (strict)"("NumText.Text"=w349) -> ()  [unwired: 2 in, 2 out]
                          }
                        }
                      }
                      frame True {
                        n139 = stacked-sequence {
                          seq-local: [w417 _] -> [_ w420]
                          tunnel: [w416 _] -> w362
                          frame #0 {
                            n140 = property on="initial time" class="DigNum (strict)"() -> ("NumText.Text"=w419:string)  [unwired: 2 in, 2 out]
                            n141 = Decimal String To Number(string=w419) -> (number=w418:i32)  [unwired: 2 in, 1 out]
                            n142 = Tick Count (ms)() -> (millisecond timer value=w417:u32)
                            n143 = Subtract(x=w417, y=w418) -> (x-y=w416:u32)
                          }
                          frame #1 {
                            n144 = Number To Decimal String(number=w420) -> (decimal integer string=w421:string)  [unwired: 1 in]
                            n145 = property on="initial time" class="DigNum (strict)"("NumText.Text"=w421) -> ()  [unwired: 2 in, 2 out]
                          }
                        }
                        n146 = Increment(x=w355) -> (x+1=w367:i32)
                        n147 = Increment(x=w369) -> (x+1=w368:i32)
                        n148 = Current VI's Path() -> (path=w365:path)
                        n149 = Strip Path(path=w365) -> (stripped path=w364:path)  [unwired: 1 out]
                        n150 = Build Path(base path=w364, name or relative path="successful_hit.wav") -> (appended path=w366:path)
                        n151 = call <vilib>:"Play Sound File.vi"("path"=w366) -> ()  [unwired: 9 in, 2 out]
                        n152 = stacked-sequence {
                          tunnel: w361 -> [w372 w384 w395 w405 w414]
                          tunnel: w362 -> [_ w382 _ _ _]
                          tunnel: w360 -> [_ _ w392 _ _]
                          tunnel: [_ _ w393 _ _] -> w359
                          tunnel: w358 -> [_ _ w394 _ _]
                          tunnel: w357 -> [_ w378 _ _ _]
                          tunnel: w353 -> [w374 _ _ _ _]
                          tunnel: [dbl[][] [] _ _ _ _] -> w352
                          frame #0 {
                            n153 = call-poly <vilib>:"Write To Spreadsheet File.vi"("append to file? (new file:F)"=TRUE, "2D data"=w374, "file path (dialog if empty)"=w372) -> ()  [unwired: 5 in, 1 out]
                          }
                          frame #1 {
                            n154 = Greater?(x=w378, y=u32 10000 ("element")) -> (0:w380:bool)
                            n155 = Select(t=1, s=w380, f=w378) -> (s? t:f=w376:i32)
                            n156 = Build Array(w382, w376, u32 0 ("element")) -> (w383:u32[])
                            n157 = call-poly <vilib>:"Write To Spreadsheet File.vi"("append to file? (new file:F)"=TRUE, "1D data"=w383, "file path (dialog if empty)"=w384) -> ()  [unwired: 5 in, 1 out]
                          }
                          frame #2 {
                            w393 = u32 0 ("element")
                            n158 = call "3D_to_Pixels.vi"("Distance_3D"=w392) -> ("Distance_pixels"=w391:dbl)  [unwired: 11 in, 3 out]
                            n159 = Decrement(x=w394) -> (x-1=w387:u32)
                            n160 = Greater?(x=w387, y=u32 10000 ("element")) -> (0:w390:bool)
                            n161 = Select(t=1, s=w390, f=w387) -> (s? t:f=w386:u32)
                            n162 = Build Array(w391, w386, w393) -> (w397:dbl[])
                            n163 = call-poly <vilib>:"Write To Spreadsheet File.vi"("append to file? (new file:F)"=TRUE, "1D data"=w397, "file path (dialog if empty)"=w395) -> ()  [unwired: 5 in, 1 out]
                          }
                          frame #3 {
                            n164 = call "3D_to_Pixels.vi"("X_3D"=-0.8 ("element"), "Y_3D"=-0.8 ("element"), "Z_3D"=0.8 ("element")) -> ("X_pixels"=w402:dbl, "Y_pixels"=w403:dbl, "Z_pixels"=w404:dbl)  [unwired: 9 in, 1 out]
                            n165 = Build Array(w402, w403, w404) -> (w401:dbl[])
                            n166 = call-poly <vilib>:"Write To Spreadsheet File.vi"("append to file? (new file:F)"=TRUE, "1D data"=w401, "file path (dialog if empty)"=w405) -> ()  [unwired: 5 in, 1 out]
                          }
                          frame #4 {
                            n167 = call "3D_to_Pixels.vi"("X_3D"=0.8 ("element"), "Y_3D"=0.8 ("element"), "Z_3D"=-0.8 ("element")) -> ("X_pixels"=w411:dbl, "Y_pixels"=w412:dbl, "Z_pixels"=w413:dbl)  [unwired: 9 in, 1 out]
                            n168 = Build Array(w411, w412, w413) -> (w410:dbl[])
                            n169 = call-poly <vilib>:"Write To Spreadsheet File.vi"("append to file? (new file:F)"=TRUE, "1D data"=w410, "file path (dialog if empty)"=w414) -> ()  [unwired: 5 in, 1 out]
                          }
                        }
                      }
                    }
                  }
                }
              }
              frame 1 {
                n170 = Unbundle(w424) -> ("X_3D"=w439:dbl, "Y_3D"=w438:dbl, "Z_3D"=w437:dbl)
                n171 = call "3D_Session_Data.vi"("Session"=w423) -> ("Radius"=w422:sgl, "min"=w427:dbl, "max"=w426:dbl)  [unwired: 8 in]
                n172 = Less Or Equal?(x=w439, y=w426) -> (x <= y?=w435:bool)
                n173 = Greater Or Equal?(x=w439, y=w427) -> (x >= y?=w436:bool)
                n174 = Less Or Equal?(x=w437, y=w426) -> (x <= y?=w431:bool)
                n175 = Greater Or Equal?(x=w437, y=w427) -> (x >= y?=w432:bool)
                n176 = Negate(x=w426) -> (-x=w429:dbl)
                n177 = Negate(x=w427) -> (-x=w428:dbl)
                n178 = Greater Or Equal?(x=w438, y=w429) -> (x >= y?=w434:bool)
                n179 = Less Or Equal?(x=w438, y=w428) -> (x <= y?=w433:bool)
                n180 = Build Array(w436, w435, w434, w433, w432, w431) -> (w430:bool[])
                n181 = And Array Elements(Boolean array=w430) -> (logical AND=w425:bool)
                n182 = case shown="True" w425 {
                  tunnel: [T12[] [{"Red"=0.0, "Green"=0.0, "Blue"=0.545, "Alpha"=0.8}, {"Red"=0.0, "Green"=0.0, "Blue"=0.545, "Alpha"=0.8}, {"Red"=0.0, "Green"=0.0, "Blue"=0.545, "Alpha"=0.8}, {"Red"=0.0, "Green"=0.0, "Blue"=0.545, "Alpha"=0.8}, {"Red"=0.0, "Green"=0.0, "Blue"=0.545, "Alpha"=0.8}, {"Red"=0.0, "Green"=0.0, "Blue"=0.545, "Alpha"=0.8}, {"Red"=0.0, "Green"=0.0, "Blue"=0.545, "Alpha"=0.8}, {"Red"=0.0, "Green"=1.0, "Blue"=1.0, "Alpha"=0.8}] ("Array") w501] -> w456
                  tunnel: [T11 {"Red"=1.0, "Green"=0.0, "Blue"=0.0, "Alpha"=1.0} ("Color") w500] -> w455
                  tunnel: w443 -> [w460 w499]
                  tunnel: w454 -> [w469 w498]
                  tunnel: [w469 w497] -> w453
                  tunnel: w452 -> [w468 w496]
                  tunnel: [w468 w495] -> w451
                  tunnel: w450 -> [_ w494]
                  tunnel: w422 -> [_ w493]
                  tunnel: [w467 w492] -> w449
                  tunnel: w448 -> [w467 w491]
                  tunnel: w447 -> [w464 w488]
                  tunnel: w446 -> [w463 w490]
                  tunnel: [w462 w488] -> w445
                  tunnel: [w461 w489] -> w444
                  tunnel: w424 -> [w459 w487]
                  tunnel: [w459 w486] -> w442
                  tunnel: [w458 w485] -> w441
                  tunnel: w440 -> [w458 w484]
                  frame False {
                    n183 = case shown="False" w460 {
                      tunnel: w464 -> [w471 w483]
                      tunnel: [w472 w482] -> w462
                      tunnel: w463 -> [w474 w481]
                      tunnel: [w473 w481] -> w461
                      frame False {
                        n184 = Greater Than 0?(x=w471) -> (x > 0?=w475:bool)
                        n185 = case shown="False" w475 {
                          tunnel: w474 -> [w477 w480]
                          tunnel: [w477 w479] -> w473
                          tunnel: w471 -> [w476 _]
                          tunnel: [w476 0 ("missed hits")] -> w472
                          frame False {
                          }
                          frame True {
                            n186 = Increment(x=w480) -> (x+1=w479:i32)
                          }
                        }
                      }
                      frame True {
                        n187 = Increment(x=w483) -> (x+1=w482:i32)
                      }
                    }
                    n188 = Number To Decimal String(number=0) -> (decimal integer string=w466:string)  [unwired: 1 in]
                    n189 = property on="initial time 2" class="DigNum (strict)"("NumText.Text"=w466) -> ()  [unwired: 2 in, 2 out]
                  }
                  frame True {
                    n190 = case shown="True" w499 {
                      tunnel: [T12[] [{"Red"=0.0, "Green"=0.0, "Blue"=0.545, "Alpha"=0.8}, {"Red"=0.0, "Green"=0.0, "Blue"=0.545, "Alpha"=0.8}, {"Red"=0.0, "Green"=0.0, "Blue"=0.545, "Alpha"=0.8}, {"Red"=0.0, "Green"=0.0, "Blue"=0.545, "Alpha"=0.8}, {"Red"=0.0, "Green"=0.0, "Blue"=0.545, "Alpha"=0.8}, {"Red"=0.0, "Green"=0.0, "Blue"=0.545, "Alpha"=0.8}, {"Red"=0.0, "Green"=0.0, "Blue"=0.545, "Alpha"=0.8}, {"Red"=0.0, "Green"=0.8, "Blue"=0.0, "Alpha"=0.8}] ("Array") T12[] [{"Red"=0.0, "Green"=0.0, "Blue"=0.545, "Alpha"=0.8}, {"Red"=0.0, "Green"=0.0, "Blue"=0.545, "Alpha"=0.8}, {"Red"=0.0, "Green"=0.0, "Blue"=0.545, "Alpha"=0.8}, {"Red"=0.0, "Green"=0.0, "Blue"=0.545, "Alpha"=0.8}, {"Red"=0.0, "Green"=0.0, "Blue"=0.545, "Alpha"=0.8}, {"Red"=0.0, "Green"=0.0, "Blue"=0.545, "Alpha"=0.8}, {"Red"=0.0, "Green"=0.0, "Blue"=0.545, "Alpha"=0.8}, {"Red"=1.0, "Green"=1.0, "Blue"=0.0, "Alpha"=0.8}] ("Array")] -> w501
                      tunnel: [T11 {"Red"=0.0, "Green"=0.8, "Blue"=0.0, "Alpha"=1.0} ("Color") T11 {"Red"=1.0, "Green"=1.0, "Blue"=0.0, "Alpha"=1.0} ("Color")] -> w500
                      tunnel: w498 -> [w512 w537]
                      tunnel: [w512 w536] -> w497
                      tunnel: w496 -> [w511 w524]
                      tunnel: [w511 w535] -> w495
                      tunnel: w494 -> [_ w530]
                      tunnel: w493 -> [_ w528]
                      tunnel: [w507 w527] -> w492
                      tunnel: w491 -> [w506 w526]
                      tunnel: w490 -> [w505 w523]
                      tunnel: [w505 0 ("x")] -> w489
                      tunnel: w487 -> [w504 _]
                      tunnel: [w504 cluster{dbl, dbl, "y":dbl} {0.8, -0.8, "y"=-0.8}] -> w486
                      tunnel: [w503 w521] -> w485
                      tunnel: w484 -> [w503 w520]
                      frame False {
                        n191 = property on="initial time 2" class="DigNum (strict)"() -> ("NumText.Text"=w509:string)  [unwired: 2 in, 2 out]
                        n192 = Decimal String To Number(string=w509) -> (number=w508:i32)  [unwired: 2 in, 1 out]
                        n193 = Equal To 0?(x=w508) -> (x = 0?=w510:bool)
                        n194 = case shown="False" w510 {
                          tunnel: w506 -> [w514 w518]
                          tunnel: [w514 w517] -> w507
                          frame False {
                          }
                          frame True {
                            n195 = Increment(x=w518) -> (x+1=w517:u32)
                            n196 = Number To Decimal String(number=1) -> (decimal integer string=w516:string)  [unwired: 1 in]
                            n197 = property on="initial time 2" class="DigNum (strict)"("NumText.Text"=w516) -> ()  [unwired: 2 in, 2 out]
                          }
                        }
                      }
                      frame True {
                        n198 = stacked-sequence {
                          seq-local: [w584 _] -> [_ w587]
                          tunnel: [w583 _] -> w529
                          frame #0 {
                            n199 = property on="initial time" class="DigNum (strict)"() -> ("NumText.Text"=w586:string)  [unwired: 2 in, 2 out]
                            n200 = Decimal String To Number(string=w586) -> (number=w585:i32)  [unwired: 2 in, 1 out]
                            n201 = Tick Count (ms)() -> (millisecond timer value=w584:u32)
                            n202 = Subtract(x=w584, y=w585) -> (x-y=w583:u32)
                          }
                          frame #1 {
                            n203 = Number To Decimal String(number=w587) -> (decimal integer string=w588:string)  [unwired: 1 in]
                            n204 = property on="initial time" class="DigNum (strict)"("NumText.Text"=w588) -> ()  [unwired: 2 in, 2 out]
                          }
                        }
                        n205 = Increment(x=w524) -> (x+1=w535:i32)
                        n206 = Increment(x=w537) -> (x+1=w536:i32)
                        n207 = Current VI's Path() -> (path=w533:path)
                        n208 = Strip Path(path=w533) -> (stripped path=w532:path)  [unwired: 1 out]
                        n209 = Build Path(base path=w532, name or relative path="successful_hit.wav") -> (appended path=w534:path)
                        n210 = call <vilib>:"Play Sound File.vi"("path"=w534) -> ()  [unwired: 9 in, 2 out]
                        n211 = stacked-sequence {
                          tunnel: w530 -> [w539 w551 w562 w572 w581]
                          tunnel: w529 -> [_ w549 _ _ _]
                          tunnel: w528 -> [_ _ w559 _ _]
                          tunnel: [_ _ w560 _ _] -> w527
                          tunnel: w526 -> [_ _ w561 _ _]
                          tunnel: w523 -> [_ w544 _ _ _]
                          tunnel: [dbl[][] [] _ _ _ _] -> w521
                          tunnel: w520 -> [w541 _ _ _ _]
                          frame #0 {
                            n212 = call-poly <vilib>:"Write To Spreadsheet File.vi"("append to file? (new file:F)"=TRUE, "2D data"=w541, "file path (dialog if empty)"=w539) -> ()  [unwired: 5 in, 1 out]
                          }
                          frame #1 {
                            n213 = Greater?(x=w544, y=u32 10000 ("element")) -> (0:w547:bool)
                            n214 = Select(t=1, s=w547, f=w544) -> (s? t:f=w543:i32)
                            n215 = Build Array(w549, w543, u32 0 ("element")) -> (w550:u32[])
                            n216 = call-poly <vilib>:"Write To Spreadsheet File.vi"("append to file? (new file:F)"=TRUE, "1D data"=w550, "file path (dialog if empty)"=w551) -> ()  [unwired: 5 in, 1 out]
                          }
                          frame #2 {
                            w560 = u32 0 ("element")
                            n217 = call "3D_to_Pixels.vi"("Distance_3D"=w559) -> ("Distance_pixels"=w558:dbl)  [unwired: 11 in, 3 out]
                            n218 = Decrement(x=w561) -> (x-1=w554:u32)
                            n219 = Greater?(x=w554, y=u32 10000 ("element")) -> (0:w557:bool)
                            n220 = Select(t=1, s=w557, f=w554) -> (s? t:f=w553:u32)
                            n221 = Build Array(w558, w553, w560) -> (w564:dbl[])
                            n222 = call-poly <vilib>:"Write To Spreadsheet File.vi"("append to file? (new file:F)"=TRUE, "1D data"=w564, "file path (dialog if empty)"=w562) -> ()  [unwired: 5 in, 1 out]
                          }
                          frame #3 {
                            n223 = call "3D_to_Pixels.vi"("X_3D"=-0.8 ("element"), "Y_3D"=0.8 ("element"), "Z_3D"=-0.8 ("element")) -> ("X_pixels"=w569:dbl, "Y_pixels"=w570:dbl, "Z_pixels"=w571:dbl)  [unwired: 9 in, 1 out]
                            n224 = Build Array(w569, w570, w571) -> (w568:dbl[])
                            n225 = call-poly <vilib>:"Write To Spreadsheet File.vi"("append to file? (new file:F)"=TRUE, "1D data"=w568, "file path (dialog if empty)"=w572) -> ()  [unwired: 5 in, 1 out]
                          }
                          frame #4 {
                            n226 = call "3D_to_Pixels.vi"("X_3D"=0.8 ("element"), "Y_3D"=-0.8 ("element"), "Z_3D"=0.8 ("element")) -> ("X_pixels"=w580:dbl, "Y_pixels"=w579:dbl, "Z_pixels"=w578:dbl)  [unwired: 9 in, 1 out]
                            n227 = Build Array(w580, w579, w578) -> (w577:dbl[])
                            n228 = call-poly <vilib>:"Write To Spreadsheet File.vi"("append to file? (new file:F)"=TRUE, "1D data"=w577, "file path (dialog if empty)"=w581) -> ()  [unwired: 5 in, 1 out]
                          }
                        }
                      }
                    }
                  }
                }
              }
              frame 2 {
                n229 = Unbundle(w591) -> ("X_3D"=w606:dbl, "Y_3D"=w605:dbl, "Z_3D"=w604:dbl)
                n230 = call "3D_Session_Data.vi"("Session"=w590) -> ("Radius"=w589:sgl, "min"=w594:dbl, "max"=w593:dbl)  [unwired: 8 in]
                n231 = Less Or Equal?(x=w605, y=w593) -> (x <= y?=w600:bool)
                n232 = Greater Or Equal?(x=w605, y=w594) -> (x >= y?=w601:bool)
                n233 = Less Or Equal?(x=w604, y=w593) -> (x <= y?=w598:bool)
                n234 = Greater Or Equal?(x=w604, y=w594) -> (x >= y?=w599:bool)
                n235 = Negate(x=w593) -> (-x=w596:dbl)
                n236 = Negate(x=w594) -> (-x=w595:dbl)
                n237 = Greater Or Equal?(x=w606, y=w596) -> (x >= y?=w603:bool)
                n238 = Less Or Equal?(x=w606, y=w595) -> (x <= y?=w602:bool)
                n239 = Build Array(w603, w602, w601, w600, w599, w598) -> (w597:bool[])
                n240 = And Array Elements(Boolean array=w597) -> (logical AND=w592:bool)
                n241 = case shown="True" w592 {
                  tunnel: [T12[] [{"Red"=0.0, "Green"=0.0, "Blue"=0.545, "Alpha"=0.8}, {"Red"=0.0, "Green"=0.0, "Blue"=0.545, "Alpha"=0.8}, {"Red"=0.0, "Green"=0.0, "Blue"=0.545, "Alpha"=0.8}, {"Red"=0.0, "Green"=0.0, "Blue"=0.545, "Alpha"=0.8}, {"Red"=0.0, "Green"=1.0, "Blue"=1.0, "Alpha"=0.8}, {"Red"=0.0, "Green"=0.0, "Blue"=0.545, "Alpha"=0.8}, {"Red"=0.0, "Green"=0.0, "Blue"=0.545, "Alpha"=0.8}, {"Red"=0.0, "Green"=0.0, "Blue"=0.545, "Alpha"=0.8}] ("Array") w668] -> w623
                  tunnel: [T11 {"Red"=1.0, "Green"=0.0, "Blue"=0.0, "Alpha"=1.0} ("Color") w667] -> w622
                  tunnel: w621 -> [w627 w666]
                  tunnel: w620 -> [w636 w665]
                  tunnel: [w636 w664] -> w619
                  tunnel: w618 -> [w635 w663]
                  tunnel: [w635 w662] -> w617
                  tunnel: w616 -> [_ w661]
                  tunnel: w589 -> [_ w660]
                  tunnel: [w634 w659] -> w615
                  tunnel: w614 -> [w634 w658]
                  tunnel: w613 -> [w631 w655]
                  tunnel: w612 -> [w630 w657]
                  tunnel: [w629 w655] -> w611
                  tunnel: [w628 w656] -> w610
                  tunnel: w591 -> [w626 w654]
                  tunnel: [w626 w653] -> w609
                  tunnel: w608 -> [w625 w652]
                  tunnel: [w625 w651] -> w607
                  frame False {
                    n242 = case shown="True" w627 {
                      tunnel: w631 -> [w638 w650]
                      tunnel: [w639 w649] -> w629
                      tunnel: w630 -> [w641 w648]
                      tunnel: [w640 w648] -> w628
                      frame False {
                        n243 = Greater Than 0?(x=w638) -> (x > 0?=w642:bool)
                        n244 = case shown="False" w642 {
                          tunnel: w641 -> [w644 w647]
                          tunnel: [w644 w646] -> w640
                          tunnel: w638 -> [w643 _]
                          tunnel: [w643 0 ("y")] -> w639
                          frame False {
                          }
                          frame True {
                            n245 = Increment(x=w647) -> (x+1=w646:i32)
                          }
                        }
                      }
                      frame True {
                        n246 = Increment(x=w650) -> (x+1=w649:i32)
                      }
                    }
                    n247 = Number To Decimal String(number=0) -> (decimal integer string=w633:string)  [unwired: 1 in]
                    n248 = property on="initial time 2" class="DigNum (strict)"("NumText.Text"=w633) -> ()  [unwired: 2 in, 2 out]
                  }
                  frame True {
                    n249 = case shown="True" w666 {
                      tunnel: [T12[] [{"Red"=0.0, "Green"=0.0, "Blue"=0.545, "Alpha"=0.8}, {"Red"=0.0, "Green"=0.0, "Blue"=0.545, "Alpha"=0.8}, {"Red"=0.0, "Green"=0.0, "Blue"=0.545, "Alpha"=0.8}, {"Red"=0.0, "Green"=0.0, "Blue"=0.545, "Alpha"=0.8}, {"Red"=0.0, "Green"=0.8, "Blue"=0.0, "Alpha"=0.8}, {"Red"=0.0, "Green"=0.0, "Blue"=0.545, "Alpha"=0.8}, {"Red"=0.0, "Green"=0.0, "Blue"=0.545, "Alpha"=0.8}, {"Red"=0.0, "Green"=0.0, "Blue"=0.545, "Alpha"=0.8}] ("Array") T12[] [{"Red"=0.0, "Green"=0.0, "Blue"=0.545, "Alpha"=0.8}, {"Red"=0.0, "Green"=0.0, "Blue"=0.545, "Alpha"=0.8}, {"Red"=0.0, "Green"=0.0, "Blue"=0.545, "Alpha"=0.8}, {"Red"=0.0, "Green"=0.0, "Blue"=0.545, "Alpha"=0.8}, {"Red"=1.0, "Green"=1.0, "Blue"=0.0, "Alpha"=0.8}, {"Red"=0.0, "Green"=0.0, "Blue"=0.545, "Alpha"=0.8}, {"Red"=0.0, "Green"=0.0, "Blue"=0.545, "Alpha"=0.8}, {"Red"=0.0, "Green"=0.0, "Blue"=0.545, "Alpha"=0.8}] ("Array")] -> w668
                      tunnel: [T11 {"Red"=0.0, "Green"=0.8, "Blue"=0.0, "Alpha"=1.0} ("Color") T11 {"Red"=1.0, "Green"=1.0, "Blue"=0.0, "Alpha"=1.0} ("Color")] -> w667
                      tunnel: w665 -> [w679 w704]
                      tunnel: [w679 w703] -> w664
                      tunnel: w663 -> [w678 w702]
                      tunnel: [w678 w701] -> w662
                      tunnel: w661 -> [_ w695]
                      tunnel: w660 -> [_ w694]
                      tunnel: [w673 w693] -> w659
                      tunnel: w658 -> [w674 w692]
                      tunnel: w657 -> [w672 w691]
                      tunnel: [w672 0 ("missed clicks")] -> w656
                      tunnel: w654 -> [w671 _]
                      tunnel: [w671 cluster{dbl, dbl, "y":dbl} {0.8, 0.8, "y"=0.8}] -> w653
                      tunnel: w652 -> [w670 w688]
                      tunnel: [w670 w687] -> w651
                      frame False {
                        n250 = property on="initial time 2" class="DigNum (strict)"() -> ("NumText.Text"=w676:string)  [unwired: 2 in, 2 out]
                        n251 = Decimal String To Number(string=w676) -> (number=w675:i32)  [unwired: 2 in, 1 out]
                        n252 = Equal To 0?(x=w675) -> (x = 0?=w677:bool)
                        n253 = case shown="True" w677 {
                          tunnel: w674 -> [w681 w685]
                          tunnel: [w681 w684] -> w673
                          frame False {
                          }
                          frame True {
                            n254 = Increment(x=w685) -> (x+1=w684:u32)
                            n255 = Number To Decimal String(number=1) -> (decimal integer string=w683:string)  [unwired: 1 in]
                            n256 = property on="initial time 2" class="DigNum (strict)"("NumText.Text"=w683) -> ()  [unwired: 2 in, 2 out]
                          }
                        }
                      }
                      frame True {
                        n257 = stacked-sequence {
                          seq-local: [w751 _] -> [_ w754]
                          tunnel: [w750 _] -> w696
                          frame #0 {
                            n258 = property on="initial time" class="DigNum (strict)"() -> ("NumText.Text"=w753:string)  [unwired: 2 in, 2 out]
                            n259 = Decimal String To Number(string=w753) -> (number=w752:i32)  [unwired: 2 in, 1 out]
                            n260 = Tick Count (ms)() -> (millisecond timer value=w751:u32)
                            n261 = Subtract(x=w751, y=w752) -> (x-y=w750:u32)
                          }
                          frame #1 {
                            n262 = Number To Decimal String(number=w754) -> (decimal integer string=w755:string)  [unwired: 1 in]
                            n263 = property on="initial time" class="DigNum (strict)"("NumText.Text"=w755) -> ()  [unwired: 2 in, 2 out]
                          }
                        }
                        n264 = Increment(x=w702) -> (x+1=w701:i32)
                        n265 = Increment(x=w704) -> (x+1=w703:i32)
                        n266 = Current VI's Path() -> (path=w699:path)
                        n267 = Strip Path(path=w699) -> (stripped path=w698:path)  [unwired: 1 out]
                        n268 = Build Path(base path=w698, name or relative path="successful_hit.wav") -> (appended path=w700:path)
                        n269 = call <vilib>:"Play Sound File.vi"("path"=w700) -> ()  [unwired: 9 in, 2 out]
                        n270 = stacked-sequence {
                          tunnel: w695 -> [w706 w718 w729 w739 w748]
                          tunnel: w696 -> [_ w716 _ _ _]
                          tunnel: w694 -> [_ _ w725 _ _]
                          tunnel: [_ _ w727 _ _] -> w693
                          tunnel: w692 -> [_ _ w728 _ _]
                          tunnel: w691 -> [_ w711 _ _ _]
                          tunnel: w688 -> [w708 _ _ _ _]
                          tunnel: [dbl[][] [] _ _ _ _] -> w687
                          frame #0 {
                            n271 = call-poly <vilib>:"Write To Spreadsheet File.vi"("append to file? (new file:F)"=TRUE, "2D data"=w708, "file path (dialog if empty)"=w706) -> ()  [unwired: 5 in, 1 out]
                          }
                          frame #1 {
                            n272 = Greater?(x=w711, y=u32 10000 ("element")) -> (0:w714:bool)
                            n273 = Select(t=1, s=w714, f=w711) -> (s? t:f=w710:i32)
                            n274 = Build Array(w716, w710, u32 0 ("element")) -> (w717:u32[])
                            n275 = call-poly <vilib>:"Write To Spreadsheet File.vi"("append to file? (new file:F)"=TRUE, "1D data"=w717, "file path (dialog if empty)"=w718) -> ()  [unwired: 5 in, 1 out]
                          }
                          frame #2 {
                            w727 = u32 0 ("element")
                            n276 = call "3D_to_Pixels.vi"("Distance_3D"=w725) -> ("Distance_pixels"=w726:dbl)  [unwired: 11 in, 3 out]
                            n277 = Decrement(x=w728) -> (x-1=w721:u32)
                            n278 = Greater?(x=w721, y=u32 10000 ("element")) -> (0:w724:bool)
                            n279 = Select(t=1, s=w724, f=w721) -> (s? t:f=w720:u32)
                            n280 = Build Array(w726, w720, w727) -> (w730:dbl[])
                            n281 = call-poly <vilib>:"Write To Spreadsheet File.vi"("append to file? (new file:F)"=TRUE, "1D data"=w730, "file path (dialog if empty)"=w729) -> ()  [unwired: 5 in, 1 out]
                          }
                          frame #3 {
                            n282 = call "3D_to_Pixels.vi"("X_3D"=0.8 ("element"), "Y_3D"=-0.8 ("element"), "Z_3D"=-0.8 ("element")) -> ("X_pixels"=w738:dbl, "Y_pixels"=w737:dbl, "Z_pixels"=w736:dbl)  [unwired: 9 in, 1 out]
                            n283 = Build Array(w738, w737, w736) -> (w735:dbl[])
                            n284 = call-poly <vilib>:"Write To Spreadsheet File.vi"("append to file? (new file:F)"=TRUE, "1D data"=w735, "file path (dialog if empty)"=w739) -> ()  [unwired: 5 in, 1 out]
                          }
                          frame #4 {
                            n285 = call "3D_to_Pixels.vi"("X_3D"=-0.8 ("element"), "Y_3D"=0.8 ("element"), "Z_3D"=0.8 ("element")) -> ("X_pixels"=w747:dbl, "Y_pixels"=w746:dbl, "Z_pixels"=w745:dbl)  [unwired: 9 in, 1 out]
                            n286 = Build Array(w747, w746, w745) -> (w744:dbl[])
                            n287 = call-poly <vilib>:"Write To Spreadsheet File.vi"("append to file? (new file:F)"=TRUE, "1D data"=w744, "file path (dialog if empty)"=w748) -> ()  [unwired: 5 in, 1 out]
                          }
                        }
                      }
                    }
                  }
                }
              }
              frame 3 {
                n288 = call "3D_Session_Data.vi"("Session"=w756) -> ("Radius"=w759:sgl, "min"=w763:dbl, "max"=w757:dbl)  [unwired: 8 in]
                n289 = Unbundle(w758) -> ("X_3D"=w773:dbl, "Y_3D"=w772:dbl, "Z_3D"=w771:dbl)
                n290 = Negate(x=w757) -> (-x=w762:dbl)
                n291 = Negate(x=w763) -> (-x=w761:dbl)
                n292 = Greater Or Equal?(x=w773, y=w762) -> (x >= y?=w770:bool)
                n293 = Greater Or Equal?(x=w772, y=w762) -> (x >= y?=w768:bool)
                n294 = Greater Or Equal?(x=w771, y=w762) -> (x >= y?=w766:bool)
                n295 = Less Or Equal?(x=w773, y=w761) -> (x <= y?=w769:bool)
                n296 = Less Or Equal?(x=w772, y=w761) -> (x <= y?=w767:bool)
                n297 = Less Or Equal?(x=w771, y=w761) -> (x <= y?=w765:bool)
                n298 = Build Array(w770, w769, w768, w767, w766, w765) -> (w764:bool[])
                n299 = And Array Elements(Boolean array=w764) -> (logical AND=w760:bool)
                n300 = case shown="True" w760 {
                  tunnel: [T12[] [{"Red"=0.0, "Green"=0.0, "Blue"=0.545, "Alpha"=0.8}, {"Red"=0.0, "Green"=0.0, "Blue"=0.545, "Alpha"=0.8}, {"Red"=0.0, "Green"=0.0, "Blue"=0.545, "Alpha"=0.8}, {"Red"=0.0, "Green"=1.0, "Blue"=1.0, "Alpha"=0.8}, {"Red"=0.0, "Green"=0.0, "Blue"=0.545, "Alpha"=0.8}, {"Red"=0.0, "Green"=0.0, "Blue"=0.545, "Alpha"=0.8}, {"Red"=0.0, "Green"=0.0, "Blue"=0.545, "Alpha"=0.8}, {"Red"=0.0, "Green"=0.0, "Blue"=0.545, "Alpha"=0.8}] ("Array") w835] -> w790
                  tunnel: [T11 {"Red"=1.0, "Green"=0.0, "Blue"=0.0, "Alpha"=1.0} ("Color") w834] -> w789
                  tunnel: w788 -> [w794 w833]
                  tunnel: w787 -> [w803 w832]
                  tunnel: [w803 w831] -> w786
                  tunnel: w785 -> [w802 w830]
                  tunnel: [w802 w829] -> w784
                  tunnel: w783 -> [_ w828]
                  tunnel: w759 -> [_ w827]
                  tunnel: [w801 w826] -> w782
                  tunnel: w781 -> [w801 w825]
                  tunnel: w780 -> [w798 w824]
                  tunnel: w779 -> [w797 w823]
                  tunnel: [w796 w824] -> w778
                  tunnel: [w795 w822] -> w777
                  tunnel: w758 -> [w793 w821]
                  tunnel: [w793 w820] -> w776
                  tunnel: w775 -> [w792 w819]
                  tunnel: [w792 w818] -> w774
                  frame False {
                    n301 = case shown="False" w794 {
                      tunnel: w798 -> [w806 w817]
                      tunnel: [w805 w816] -> w796
                      tunnel: w797 -> [w808 w815]
                      tunnel: [w807 w815] -> w795
                      frame False {
                        n302 = Equal To 0?(x=w806) -> (x = 0?=w809:bool)
                        n303 = case shown="True" w809 {
                          tunnel: w808 -> [w811 w814]
                          tunnel: [w811 w813] -> w807
                          tunnel: w806 -> [w810 _]
                          tunnel: [w810 0 ("y")] -> w805
                          frame False {
                          }
                          frame True {
                            n304 = Increment(x=w814) -> (x+1=w813:i32)
                          }
                        }
                      }
                      frame True {
                        n305 = Increment(x=w817) -> (x+1=w816:i32)
                      }
                    }
                    n306 = Number To Decimal String(number=0) -> (decimal integer string=w800:string)  [unwired: 1 in]
                    n307 = property on="initial time 2" class="DigNum (strict)"("NumText.Text"=w800) -> ()  [unwired: 2 in, 2 out]
                  }
                  frame True {
                    n308 = case shown="True" w833 {
                      tunnel: [T12[] [{"Red"=0.0, "Green"=0.0, "Blue"=0.545, "Alpha"=0.8}, {"Red"=0.0, "Green"=0.0, "Blue"=0.545, "Alpha"=0.8}, {"Red"=0.0, "Green"=0.0, "Blue"=0.545, "Alpha"=0.8}, {"Red"=0.0, "Green"=0.8, "Blue"=0.0, "Alpha"=0.8}, {"Red"=0.0, "Green"=0.0, "Blue"=0.545, "Alpha"=0.8}, {"Red"=0.0, "Green"=0.0, "Blue"=0.545, "Alpha"=0.8}, {"Red"=0.0, "Green"=0.0, "Blue"=0.545, "Alpha"=0.8}, {"Red"=0.0, "Green"=0.0, "Blue"=0.545, "Alpha"=0.8}] ("Array") T12[] [{"Red"=0.0, "Green"=0.0, "Blue"=0.545, "Alpha"=0.8}, {"Red"=0.0, "Green"=0.0, "Blue"=0.545, "Alpha"=0.8}, {"Red"=0.0, "Green"=0.0, "Blue"=0.545, "Alpha"=0.8}, {"Red"=1.0, "Green"=1.0, "Blue"=0.0, "Alpha"=0.8}, {"Red"=0.0, "Green"=0.0, "Blue"=0.545, "Alpha"=0.8}, {"Red"=0.0, "Green"=0.0, "Blue"=0.545, "Alpha"=0.8}, {"Red"=0.0, "Green"=0.0, "Blue"=0.545, "Alpha"=0.8}, {"Red"=0.0, "Green"=0.0, "Blue"=0.545, "Alpha"=0.8}] ("Array")] -> w835
                      tunnel: [T11 {"Red"=0.0, "Green"=0.8, "Blue"=0.0, "Alpha"=1.0} ("Color") T11 {"Red"=1.0, "Green"=1.0, "Blue"=0.0, "Alpha"=1.0} ("Color")] -> w834
                      tunnel: w832 -> [w846 w871]
                      tunnel: [w846 w870] -> w831
                      tunnel: w830 -> [w845 w869]
                      tunnel: [w845 w868] -> w829
                      tunnel: w828 -> [_ w862]
                      tunnel: w827 -> [_ w861]
                      tunnel: [w840 w860] -> w826
                      tunnel: w825 -> [w841 w859]
                      tunnel: w823 -> [w839 w858]
                      tunnel: [w839 0 ("y")] -> w822
                      tunnel: w821 -> [w838 _]
                      tunnel: [w838 cluster{dbl, dbl, "y":dbl} {-0.8, -0.8, "y"=-0.8}] -> w820
                      tunnel: w819 -> [w837 w855]
                      tunnel: [w837 w854] -> w818
                      frame False {
                        n309 = property on="initial time 2" class="DigNum (strict)"() -> ("NumText.Text"=w843:string)  [unwired: 2 in, 2 out]
                        n310 = Decimal String To Number(string=w843) -> (number=w842:i32)  [unwired: 2 in, 1 out]
                        n311 = Equal To 0?(x=w842) -> (x = 0?=w844:bool)
                        n312 = case shown="False" w844 {
                          tunnel: w841 -> [w848 w852]
                          tunnel: [w848 w851] -> w840
                          frame False {
                          }
                          frame True {
                            n313 = Increment(x=w852) -> (x+1=w851:u32)
                            n314 = Number To Decimal String(number=1) -> (decimal integer string=w850:string)  [unwired: 1 in]
                            n315 = property on="initial time 2" class="DigNum (strict)"("NumText.Text"=w850) -> ()  [unwired: 2 in, 2 out]
                          }
                        }
                      }
                      frame True {
                        n316 = stacked-sequence {
                          seq-local: [w918 _] -> [_ w921]
                          tunnel: [w917 _] -> w863
                          frame #0 {
                            n317 = property on="initial time" class="DigNum (strict)"() -> ("NumText.Text"=w920:string)  [unwired: 2 in, 2 out]
                            n318 = Decimal String To Number(string=w920) -> (number=w919:i32)  [unwired: 2 in, 1 out]
                            n319 = Tick Count (ms)() -> (millisecond timer value=w918:u32)
                            n320 = Subtract(x=w918, y=w919) -> (x-y=w917:u32)
                          }
                          frame #1 {
                            n321 = Number To Decimal String(number=w921) -> (decimal integer string=w922:string)  [unwired: 1 in]
                            n322 = property on="initial time" class="DigNum (strict)"("NumText.Text"=w922) -> ()  [unwired: 2 in, 2 out]
                          }
                        }
                        n323 = Increment(x=w869) -> (x+1=w868:i32)
                        n324 = Increment(x=w871) -> (x+1=w870:i32)
                        n325 = Current VI's Path() -> (path=w866:path)
                        n326 = Strip Path(path=w866) -> (stripped path=w865:path)  [unwired: 1 out]
                        n327 = Build Path(base path=w865, name or relative path="successful_hit.wav") -> (appended path=w867:path)
                        n328 = call <vilib>:"Play Sound File.vi"("path"=w867) -> ()  [unwired: 9 in, 2 out]
                        n329 = stacked-sequence {
                          tunnel: w862 -> [w873 w885 w896 w906 w915]
                          tunnel: w863 -> [_ w883 _ _ _]
                          tunnel: w861 -> [_ _ w893 _ _]
                          tunnel: [_ _ w894 _ _] -> w860
                          tunnel: w859 -> [_ _ w895 _ _]
                          tunnel: w858 -> [_ w878 _ _ _]
                          tunnel: w855 -> [w874 _ _ _ _]
                          tunnel: [dbl[][] [] _ _ _ _] -> w854
                          frame #0 {
                            n330 = call-poly <vilib>:"Write To Spreadsheet File.vi"("append to file? (new file:F)"=TRUE, "2D data"=w874, "file path (dialog if empty)"=w873) -> ()  [unwired: 5 in, 1 out]
                          }
                          frame #1 {
                            n331 = Greater?(x=w878, y=u32 10000 ("element")) -> (0:w881:bool)
                            n332 = Select(t=1, s=w881, f=w878) -> (s? t:f=w877:i32)
                            n333 = Build Array(w883, w877, u32 0 ("element")) -> (w884:u32[])
                            n334 = call-poly <vilib>:"Write To Spreadsheet File.vi"("append to file? (new file:F)"=TRUE, "1D data"=w884, "file path (dialog if empty)"=w885) -> ()  [unwired: 5 in, 1 out]
                          }
                          frame #2 {
                            w894 = u32 0 ("element")
                            n335 = call "3D_to_Pixels.vi"("Distance_3D"=w893) -> ("Distance_pixels"=w892:dbl)  [unwired: 11 in, 3 out]
                            n336 = Decrement(x=w895) -> (x-1=w888:u32)
                            n337 = Greater?(x=w888, y=u32 10000 ("element")) -> (0:w891:bool)
                            n338 = Select(t=1, s=w891, f=w888) -> (s? t:f=w887:u32)
                            n339 = Build Array(w892, w887, w894) -> (w897:dbl[])
                            n340 = call-poly <vilib>:"Write To Spreadsheet File.vi"("append to file? (new file:F)"=TRUE, "1D data"=w897, "file path (dialog if empty)"=w896) -> ()  [unwired: 5 in, 1 out]
                          }
                          frame #3 {
                            n341 = call "3D_to_Pixels.vi"("X_3D"=0.8 ("element"), "Y_3D"=0.8 ("element"), "Z_3D"=0.8 ("element")) -> ("X_pixels"=w905:dbl, "Y_pixels"=w904:dbl, "Z_pixels"=w903:dbl)  [unwired: 9 in, 1 out]
                            n342 = Build Array(w905, w904, w903) -> (w902:dbl[])
                            n343 = call-poly <vilib>:"Write To Spreadsheet File.vi"("append to file? (new file:F)"=TRUE, "1D data"=w902, "file path (dialog if empty)"=w906) -> ()  [unwired: 5 in, 1 out]
                          }
                          frame #4 {
                            n344 = call "3D_to_Pixels.vi"("X_3D"=-0.8 ("element"), "Y_3D"=-0.8 ("element"), "Z_3D"=-0.8 ("element")) -> ("X_pixels"=w914:dbl, "Y_pixels"=w913:dbl, "Z_pixels"=w912:dbl)  [unwired: 9 in, 1 out]
                            n345 = Build Array(w914, w913, w912) -> (w908:dbl[])
                            n346 = call-poly <vilib>:"Write To Spreadsheet File.vi"("append to file? (new file:F)"=TRUE, "1D data"=w908, "file path (dialog if empty)"=w915) -> ()  [unwired: 5 in, 1 out]
                          }
                        }
                      }
                    }
                  }
                }
              }
              frame 4 {
                n347 = Unbundle(w924) -> ("X_3D"=w938:dbl, "Y_3D"=w937:dbl, "Z_3D"=w936:dbl)
                n348 = call "3D_Session_Data.vi"("Session"=w925) -> ("Radius"=w923:sgl, "min"=w928:dbl, "max"=w927:dbl)  [unwired: 8 in]
                n349 = Less Or Equal?(x=w938, y=w927) -> (x <= y?=w934:bool)
                n350 = Greater Or Equal?(x=w938, y=w928) -> (x >= y?=w935:bool)
                n351 = Less Or Equal?(x=w937, y=w927) -> (x <= y?=w932:bool)
                n352 = Greater Or Equal?(x=w937, y=w928) -> (x >= y?=w933:bool)
                n353 = Less Or Equal?(x=w936, y=w927) -> (x <= y?=w930:bool)
                n354 = Greater Or Equal?(x=w936, y=w928) -> (x >= y?=w931:bool)
                n355 = Build Array(w935, w934, w933, w932, w931, w930) -> (w929:bool[])
                n356 = And Array Elements(Boolean array=w929) -> (logical AND=w926:bool)
                n357 = case shown="True" w926 {
                  tunnel: [T12[] [{"Red"=0.0, "Green"=0.0, "Blue"=0.545, "Alpha"=0.8}, {"Red"=0.0, "Green"=0.0, "Blue"=0.545, "Alpha"=0.8}, {"Red"=0.0, "Green"=1.0, "Blue"=1.0, "Alpha"=0.8}, {"Red"=0.0, "Green"=0.0, "Blue"=0.545, "Alpha"=0.8}, {"Red"=0.0, "Green"=0.0, "Blue"=0.545, "Alpha"=0.8}, {"Red"=0.0, "Green"=0.0, "Blue"=0.545, "Alpha"=0.8}, {"Red"=0.0, "Green"=0.0, "Blue"=0.545, "Alpha"=0.8}, {"Red"=0.0, "Green"=0.0, "Blue"=0.545, "Alpha"=0.8}] ("Array") w1000] -> w955
                  tunnel: [T11 {"Red"=1.0, "Green"=0.0, "Blue"=0.0, "Alpha"=1.0} ("Color") w999] -> w954
                  tunnel: w953 -> [w959 w998]
                  tunnel: w952 -> [w968 w997]
                  tunnel: [w968 w996] -> w951
                  tunnel: w950 -> [w967 w995]
                  tunnel: [w967 w994] -> w949
                  tunnel: w948 -> [_ w993]
                  tunnel: w923 -> [_ w992]
                  tunnel: [w966 w990] -> w947
                  tunnel: w946 -> [w966 w991]
                  tunnel: w945 -> [w963 w989]
                  tunnel: w944 -> [w962 w988]
                  tunnel: [w961 w989] -> w943
                  tunnel: [w960 w987] -> w942
                  tunnel: w924 -> [w958 w986]
                  tunnel: [w958 w985] -> w941
                  tunnel: w940 -> [w957 w984]
                  tunnel: [w957 w983] -> w939
                  frame False {
                    n358 = case shown="False" w959 {
                      tunnel: w963 -> [w971 w982]
                      tunnel: [w970 w981] -> w961
                      tunnel: w962 -> [w973 w980]
                      tunnel: [w972 w980] -> w960
                      frame False {
                        n359 = Greater Than 0?(x=w971) -> (x > 0?=w974:bool)
                        n360 = case shown="False" w974 {
                          tunnel: w973 -> [w976 w979]
                          tunnel: [w976 w978] -> w972
                          tunnel: w971 -> [w975 _]
                          tunnel: [w975 0 ("y")] -> w970
                          frame False {
                          }
                          frame True {
                            n361 = Increment(x=w979) -> (x+1=w978:i32)
                          }
                        }
                      }
                      frame True {
                        n362 = Increment(x=w982) -> (x+1=w981:i32)
                      }
                    }
                    n363 = Number To Decimal String(number=0) -> (decimal integer string=w965:string)  [unwired: 1 in]
                    n364 = property on="initial time 2" class="DigNum (strict)"("NumText.Text"=w965) -> ()  [unwired: 2 in, 2 out]
                  }
                  frame True {
                    n365 = case shown="True" w998 {
                      tunnel: [T12[] [{"Red"=0.0, "Green"=0.0, "Blue"=0.545, "Alpha"=0.8}, {"Red"=0.0, "Green"=0.0, "Blue"=0.545, "Alpha"=0.8}, {"Red"=0.0, "Green"=0.8, "Blue"=0.0, "Alpha"=0.8}, {"Red"=0.0, "Green"=0.0, "Blue"=0.545, "Alpha"=0.8}, {"Red"=0.0, "Green"=0.0, "Blue"=0.545, "Alpha"=0.8}, {"Red"=0.0, "Green"=0.0, "Blue"=0.545, "Alpha"=0.8}, {"Red"=0.0, "Green"=0.0, "Blue"=0.545, "Alpha"=0.8}, {"Red"=0.0, "Green"=0.0, "Blue"=0.545, "Alpha"=0.8}] ("Array") T12[] [{"Red"=0.0, "Green"=0.0, "Blue"=0.545, "Alpha"=0.8}, {"Red"=0.0, "Green"=0.0, "Blue"=0.545, "Alpha"=0.8}, {"Red"=1.0, "Green"=1.0, "Blue"=0.0, "Alpha"=0.8}, {"Red"=0.0, "Green"=0.0, "Blue"=0.545, "Alpha"=0.8}, {"Red"=0.0, "Green"=0.0, "Blue"=0.545, "Alpha"=0.8}, {"Red"=0.0, "Green"=0.0, "Blue"=0.545, "Alpha"=0.8}, {"Red"=0.0, "Green"=0.0, "Blue"=0.545, "Alpha"=0.8}, {"Red"=0.0, "Green"=0.0, "Blue"=0.545, "Alpha"=0.8}] ("Array")] -> w1000
                      tunnel: [T11 {"Red"=0.0, "Green"=0.8, "Blue"=0.0, "Alpha"=1.0} ("Color") T11 {"Red"=1.0, "Green"=1.0, "Blue"=0.0, "Alpha"=1.0} ("Color")] -> w999
                      tunnel: w997 -> [w1011 w1036]
                      tunnel: [w1011 w1035] -> w996
                      tunnel: w995 -> [w1010 w1034]
                      tunnel: [w1010 w1033] -> w994
                      tunnel: w993 -> [_ w1027]
                      tunnel: w992 -> [_ w1026]
                      tunnel: w991 -> [w1006 w1024]
                      tunnel: [w1005 w1025] -> w990
                      tunnel: w988 -> [w1004 w1023]
                      tunnel: [w1004 0 ("y")] -> w987
                      tunnel: w986 -> [w1003 _]
                      tunnel: [w1003 cluster{dbl, dbl, "y":dbl} {-0.8, 0.8, "y"=0.8}] -> w985
                      tunnel: w984 -> [w1002 w1020]
                      tunnel: [w1002 w1019] -> w983
                      frame False {
                        n366 = property on="initial time 2" class="DigNum (strict)"() -> ("NumText.Text"=w1008:string)  [unwired: 2 in, 2 out]
                        n367 = Decimal String To Number(string=w1008) -> (number=w1007:i32)  [unwired: 2 in, 1 out]
                        n368 = Equal To 0?(x=w1007) -> (x = 0?=w1009:bool)
                        n369 = case shown="True" w1009 {
                          tunnel: w1006 -> [w1013 w1017]
                          tunnel: [w1013 w1016] -> w1005
                          frame False {
                          }
                          frame True {
                            n370 = Increment(x=w1017) -> (x+1=w1016:u32)
                            n371 = Number To Decimal String(number=1) -> (decimal integer string=w1015:string)  [unwired: 1 in]
                            n372 = property on="initial time 2" class="DigNum (strict)"("NumText.Text"=w1015) -> ()  [unwired: 2 in, 2 out]
                          }
                        }
                      }
                      frame True {
                        n373 = stacked-sequence {
                          seq-local: [w1083 _] -> [_ w1086]
                          tunnel: [w1082 _] -> w1028
                          frame #0 {
                            n374 = property on="initial time" class="DigNum (strict)"() -> ("NumText.Text"=w1085:string)  [unwired: 2 in, 2 out]
                            n375 = Decimal String To Number(string=w1085) -> (number=w1084:i32)  [unwired: 2 in, 1 out]
                            n376 = Tick Count (ms)() -> (millisecond timer value=w1083:u32)
                            n377 = Subtract(x=w1083, y=w1084) -> (x-y=w1082:u32)
                          }
                          frame #1 {
                            n378 = Number To Decimal String(number=w1086) -> (decimal integer string=w1087:string)  [unwired: 1 in]
                            n379 = property on="initial time" class="DigNum (strict)"("NumText.Text"=w1087) -> ()  [unwired: 2 in, 2 out]
                          }
                        }
                        n380 = Increment(x=w1034) -> (x+1=w1033:i32)
                        n381 = Increment(x=w1036) -> (x+1=w1035:i32)
                        n382 = Current VI's Path() -> (path=w1031:path)
                        n383 = Strip Path(path=w1031) -> (stripped path=w1030:path)  [unwired: 1 out]
                        n384 = Build Path(base path=w1030, name or relative path="successful_hit.wav") -> (appended path=w1032:path)
                        n385 = call <vilib>:"Play Sound File.vi"("path"=w1032) -> ()  [unwired: 9 in, 2 out]
                        n386 = stacked-sequence {
                          tunnel: w1027 -> [w1039 w1050 w1061 w1071 w1080]
                          tunnel: w1028 -> [_ w1048 _ _ _]
                          tunnel: w1026 -> [_ _ w1059 _ _]
                          tunnel: [_ _ w1057 _ _] -> w1025
                          tunnel: w1024 -> [_ _ w1060 _ _]
                          tunnel: w1023 -> [_ w1043 _ _ _]
                          tunnel: w1020 -> [w1040 _ _ _ _]
                          tunnel: [dbl[][] [] _ _ _ _] -> w1019
                          frame #0 {
                            n387 = call-poly <vilib>:"Write To Spreadsheet File.vi"("append to file? (new file:F)"=TRUE, "2D data"=w1040, "file path (dialog if empty)"=w1039) -> ()  [unwired: 5 in, 1 out]
                          }
                          frame #1 {
                            n388 = Greater?(x=w1043, y=u32 10000 ("element")) -> (0:w1046:bool)
                            n389 = Select(t=1, s=w1046, f=w1043) -> (s? t:f=w1042:i32)
                            n390 = Build Array(w1048, w1042, u32 0 ("element")) -> (w1049:u32[])
                            n391 = call-poly <vilib>:"Write To Spreadsheet File.vi"("append to file? (new file:F)"=TRUE, "1D data"=w1049, "file path (dialog if empty)"=w1050) -> ()  [unwired: 5 in, 1 out]
                          }
                          frame #2 {
                            w1057 = u32 0 ("element")
                            n392 = call "3D_to_Pixels.vi"("Distance_3D"=w1059) -> ("Distance_pixels"=w1058:dbl)  [unwired: 11 in, 3 out]
                            n393 = Decrement(x=w1060) -> (x-1=w1053:u32)
                            n394 = Greater?(x=w1053, y=u32 10000 ("element")) -> (0:w1056:bool)
                            n395 = Select(t=1, s=w1056, f=w1053) -> (s? t:f=w1052:u32)
                            n396 = Build Array(w1058, w1052, w1057) -> (w1063:dbl[])
                            n397 = call-poly <vilib>:"Write To Spreadsheet File.vi"("append to file? (new file:F)"=TRUE, "1D data"=w1063, "file path (dialog if empty)"=w1061) -> ()  [unwired: 5 in, 1 out]
                          }
                          frame #3 {
                            n398 = call "3D_to_Pixels.vi"("X_3D"=-0.8 ("element"), "Y_3D"=-0.8 ("element"), "Z_3D"=-0.8 ("element")) -> ("X_pixels"=w1070:dbl, "Y_pixels"=w1069:dbl, "Z_pixels"=w1068:dbl)  [unwired: 9 in, 1 out]
                            n399 = Build Array(w1070, w1069, w1068) -> (w1064:dbl[])
                            n400 = call-poly <vilib>:"Write To Spreadsheet File.vi"("append to file? (new file:F)"=TRUE, "1D data"=w1064, "file path (dialog if empty)"=w1071) -> ()  [unwired: 5 in, 1 out]
                          }
                          frame #4 {
                            n401 = call "3D_to_Pixels.vi"("X_3D"=0.8 ("element"), "Y_3D"=0.8 ("element"), "Z_3D"=0.8 ("element")) -> ("X_pixels"=w1079:dbl, "Y_pixels"=w1078:dbl, "Z_pixels"=w1077:dbl)  [unwired: 9 in, 1 out]
                            n402 = Build Array(w1079, w1078, w1077) -> (w1073:dbl[])
                            n403 = call-poly <vilib>:"Write To Spreadsheet File.vi"("append to file? (new file:F)"=TRUE, "1D data"=w1073, "file path (dialog if empty)"=w1080) -> ()  [unwired: 5 in, 1 out]
                          }
                        }
                      }
                    }
                  }
                }
              }
              frame 5 {
                n404 = Unbundle(w1090) -> ("X_3D"=w1105:dbl, "Y_3D"=w1104:dbl, "Z_3D"=w1103:dbl)
                n405 = call "3D_Session_Data.vi"("Session"=w1089) -> ("Radius"=w1088:sgl, "min"=w1095:dbl, "max"=w1094:dbl)  [unwired: 8 in]
                n406 = Less Or Equal?(x=w1105, y=w1094) -> (x <= y?=w1101:bool)
                n407 = Greater Or Equal?(x=w1105, y=w1095) -> (x >= y?=w1102:bool)
                n408 = Negate(x=w1094) -> (-x=w1093:dbl)
                n409 = Negate(x=w1095) -> (-x=w1092:dbl)
                n410 = Greater Or Equal?(x=w1104, y=w1093) -> (x >= y?=w1100:bool)
                n411 = Less Or Equal?(x=w1104, y=w1092) -> (x <= y?=w1099:bool)
                n412 = Greater Or Equal?(x=w1103, y=w1093) -> (x >= y?=w1098:bool)
                n413 = Less Or Equal?(x=w1103, y=w1092) -> (x <= y?=w1097:bool)
                n414 = Build Array(w1102, w1101, w1100, w1099, w1098, w1097) -> (w1096:bool[])
                n415 = And Array Elements(Boolean array=w1096) -> (logical AND=w1091:bool)
                n416 = case shown="True" w1091 {
                  tunnel: [T12[] [{"Red"=0.0, "Green"=0.0, "Blue"=0.545, "Alpha"=0.8}, {"Red"=0.0, "Green"=0.0, "Blue"=0.545, "Alpha"=0.8}, {"Red"=0.0, "Green"=0.0, "Blue"=0.545, "Alpha"=0.8}, {"Red"=0.0, "Green"=0.0, "Blue"=0.545, "Alpha"=0.8}, {"Red"=0.0, "Green"=0.0, "Blue"=0.545, "Alpha"=0.8}, {"Red"=0.0, "Green"=1.0, "Blue"=1.0, "Alpha"=0.8}, {"Red"=0.0, "Green"=0.0, "Blue"=0.545, "Alpha"=0.8}, {"Red"=0.0, "Green"=0.0, "Blue"=0.545, "Alpha"=0.8}] ("Array") w1167] -> w1122
                  tunnel: [T11 {"Red"=1.0, "Green"=0.0, "Blue"=0.0, "Alpha"=1.0} ("Color") w1166] -> w1121
                  tunnel: w1120 -> [w1126 w1165]
                  tunnel: w1119 -> [w1135 w1164]
                  tunnel: [w1135 w1163] -> w1118
                  tunnel: w1117 -> [w1134 w1162]
                  tunnel: [w1134 w1161] -> w1116
                  tunnel: w1115 -> [_ w1160]
                  tunnel: w1088 -> [_ w1159]
                  tunnel: [w1133 w1158] -> w1114
                  tunnel: w1113 -> [w1133 w1157]
                  tunnel: w1112 -> [w1130 w1156]
                  tunnel: w1111 -> [w1129 w1155]
                  tunnel: [w1128 w1156] -> w1110
                  tunnel: [w1127 w1154] -> w1109
                  tunnel: w1090 -> [w1125 w1153]
                  tunnel: [w1125 w1152] -> w1108
                  tunnel: w1107 -> [w1124 w1151]
                  tunnel: [w1124 w1150] -> w1106
                  frame False {
                    n417 = case shown="True" w1126 {
                      tunnel: w1130 -> [w1138 w1149]
                      tunnel: [w1137 w1148] -> w1128
                      tunnel: w1129 -> [w1140 w1147]
                      tunnel: [w1139 w1147] -> w1127
                      frame False {
                        n418 = Greater Than 0?(x=w1138) -> (x > 0?=w1141:bool)
                        n419 = case shown="False" w1141 {
                          tunnel: w1140 -> [w1143 w1146]
                          tunnel: [w1143 w1145] -> w1139
                          tunnel: w1138 -> [w1142 _]
                          tunnel: [w1142 0 ("y")] -> w1137
                          frame False {
                          }
                          frame True {
                            n420 = Increment(x=w1146) -> (x+1=w1145:i32)
                          }
                        }
                      }
                      frame True {
                        n421 = Increment(x=w1149) -> (x+1=w1148:i32)
                      }
                    }
                    n422 = Number To Decimal String(number=0) -> (decimal integer string=w1132:string)  [unwired: 1 in]
                    n423 = property on="initial time 2" class="DigNum (strict)"("NumText.Text"=w1132) -> ()  [unwired: 2 in, 2 out]
                  }
                  frame True {
                    n424 = case shown="True" w1165 {
                      tunnel: [T12[] [{"Red"=0.0, "Green"=0.0, "Blue"=0.545, "Alpha"=0.8}, {"Red"=0.0, "Green"=0.0, "Blue"=0.545, "Alpha"=0.8}, {"Red"=0.0, "Green"=0.0, "Blue"=0.545, "Alpha"=0.8}, {"Red"=0.0, "Green"=0.0, "Blue"=0.545, "Alpha"=0.8}, {"Red"=0.0, "Green"=0.0, "Blue"=0.545, "Alpha"=0.8}, {"Red"=0.0, "Green"=0.8, "Blue"=0.0, "Alpha"=0.8}, {"Red"=0.0, "Green"=0.0, "Blue"=0.545, "Alpha"=0.8}, {"Red"=0.0, "Green"=0.0, "Blue"=0.545, "Alpha"=0.8}] ("Array") T12[] [{"Red"=0.0, "Green"=0.0, "Blue"=0.545, "Alpha"=0.8}, {"Red"=0.0, "Green"=0.0, "Blue"=0.545, "Alpha"=0.8}, {"Red"=0.0, "Green"=0.0, "Blue"=0.545, "Alpha"=0.8}, {"Red"=0.0, "Green"=0.0, "Blue"=0.545, "Alpha"=0.8}, {"Red"=0.0, "Green"=0.0, "Blue"=0.545, "Alpha"=0.8}, {"Red"=1.0, "Green"=1.0, "Blue"=0.0, "Alpha"=0.8}, {"Red"=0.0, "Green"=0.0, "Blue"=0.545, "Alpha"=0.8}, {"Red"=0.0, "Green"=0.0, "Blue"=0.545, "Alpha"=0.8}] ("Array")] -> w1167
                      tunnel: [T11 {"Red"=0.0, "Green"=0.8, "Blue"=0.0, "Alpha"=1.0} ("Color") T11 {"Red"=1.0, "Green"=1.0, "Blue"=0.0, "Alpha"=1.0} ("Color")] -> w1166
                      tunnel: w1164 -> [w1178 w1203]
                      tunnel: [w1178 w1202] -> w1163
                      tunnel: w1162 -> [w1177 w1201]
                      tunnel: [w1177 w1200] -> w1161
                      tunnel: w1160 -> [_ w1194]
                      tunnel: w1159 -> [_ w1193]
                      tunnel: [w1172 w1192] -> w1158
                      tunnel: w1157 -> [w1173 w1191]
                      tunnel: w1155 -> [w1171 w1190]
                      tunnel: [w1171 0 ("y")] -> w1154
                      tunnel: w1153 -> [w1170 _]
                      tunnel: [w1170 cluster{dbl, dbl, "y":dbl} {0.8, -0.8, "y"=0.8}] -> w1152
                      tunnel: w1151 -> [w1169 w1187]
                      tunnel: [w1169 w1186] -> w1150
                      frame False {
                        n425 = property on="initial time 2" class="DigNum (strict)"() -> ("NumText.Text"=w1175:string)  [unwired: 2 in, 2 out]
                        n426 = Decimal String To Number(string=w1175) -> (number=w1174:i32)  [unwired: 2 in, 1 out]
                        n427 = Equal To 0?(x=w1174) -> (x = 0?=w1176:bool)
                        n428 = case shown="False" w1176 {
                          tunnel: w1173 -> [w1180 w1184]
                          tunnel: [w1180 w1183] -> w1172
                          frame False {
                          }
                          frame True {
                            n429 = Increment(x=w1184) -> (x+1=w1183:u32)
                            n430 = Number To Decimal String(number=1) -> (decimal integer string=w1182:string)  [unwired: 1 in]
                            n431 = property on="initial time 2" class="DigNum (strict)"("NumText.Text"=w1182) -> ()  [unwired: 2 in, 2 out]
                          }
                        }
                      }
                      frame True {
                        n432 = stacked-sequence {
                          seq-local: [w1250 _] -> [_ w1253]
                          tunnel: [w1249 _] -> w1195
                          frame #0 {
                            n433 = property on="initial time" class="DigNum (strict)"() -> ("NumText.Text"=w1252:string)  [unwired: 2 in, 2 out]
                            n434 = Decimal String To Number(string=w1252) -> (number=w1251:i32)  [unwired: 2 in, 1 out]
                            n435 = Tick Count (ms)() -> (millisecond timer value=w1250:u32)
                            n436 = Subtract(x=w1250, y=w1251) -> (x-y=w1249:u32)
                          }
                          frame #1 {
                            n437 = Number To Decimal String(number=w1253) -> (decimal integer string=w1254:string)  [unwired: 1 in]
                            n438 = property on="initial time" class="DigNum (strict)"("NumText.Text"=w1254) -> ()  [unwired: 2 in, 2 out]
                          }
                        }
                        n439 = Increment(x=w1201) -> (x+1=w1200:i32)
                        n440 = Increment(x=w1203) -> (x+1=w1202:i32)
                        n441 = Current VI's Path() -> (path=w1198:path)
                        n442 = Strip Path(path=w1198) -> (stripped path=w1197:path)  [unwired: 1 out]
                        n443 = Build Path(base path=w1197, name or relative path="successful_hit.wav") -> (appended path=w1199:path)
                        n444 = call <vilib>:"Play Sound File.vi"("path"=w1199) -> ()  [unwired: 9 in, 2 out]
                        n445 = stacked-sequence {
                          tunnel: w1194 -> [w1206 w1217 w1228 w1238 w1247]
                          tunnel: w1195 -> [_ w1215 _ _ _]
                          tunnel: w1193 -> [_ _ w1225 _ _]
                          tunnel: [_ _ w1226 _ _] -> w1192
                          tunnel: w1191 -> [_ _ w1227 _ _]
                          tunnel: w1190 -> [_ w1210 _ _ _]
                          tunnel: w1187 -> [w1207 _ _ _ _]
                          tunnel: [dbl[][] [] _ _ _ _] -> w1186
                          frame #0 {
                            n446 = call-poly <vilib>:"Write To Spreadsheet File.vi"("append to file? (new file:F)"=TRUE, "2D data"=w1207, "file path (dialog if empty)"=w1206) -> ()  [unwired: 5 in, 1 out]
                          }
                          frame #1 {
                            n447 = Greater?(x=w1210, y=u32 10000 ("element")) -> (0:w1213:bool)
                            n448 = Select(t=1, s=w1213, f=w1210) -> (s? t:f=w1209:i32)
                            n449 = Build Array(w1215, w1209, u32 0 ("element")) -> (w1216:u32[])
                            n450 = call-poly <vilib>:"Write To Spreadsheet File.vi"("append to file? (new file:F)"=TRUE, "1D data"=w1216, "file path (dialog if empty)"=w1217) -> ()  [unwired: 5 in, 1 out]
                          }
                          frame #2 {
                            w1226 = u32 0 ("element")
                            n451 = call "3D_to_Pixels.vi"("Distance_3D"=w1225) -> ("Distance_pixels"=w1224:dbl)  [unwired: 11 in, 3 out]
                            n452 = Decrement(x=w1227) -> (x-1=w1220:u32)
                            n453 = Greater?(x=w1220, y=u32 10000 ("element")) -> (0:w1223:bool)
                            n454 = Select(t=1, s=w1223, f=w1220) -> (s? t:f=w1219:u32)
                            n455 = Build Array(w1224, w1219, w1226) -> (w1229:dbl[])
                            n456 = call-poly <vilib>:"Write To Spreadsheet File.vi"("append to file? (new file:F)"=TRUE, "1D data"=w1229, "file path (dialog if empty)"=w1228) -> ()  [unwired: 5 in, 1 out]
                          }
                          frame #3 {
                            n457 = call "3D_to_Pixels.vi"("X_3D"=-0.8 ("element"), "Y_3D"=0.8 ("element"), "Z_3D"=0.8 ("element")) -> ("X_pixels"=w1237:dbl, "Y_pixels"=w1236:dbl, "Z_pixels"=w1235:dbl)  [unwired: 9 in, 1 out]
                            n458 = Build Array(w1237, w1236, w1235) -> (w1231:dbl[])
                            n459 = call-poly <vilib>:"Write To Spreadsheet File.vi"("append to file? (new file:F)"=TRUE, "1D data"=w1231, "file path (dialog if empty)"=w1238) -> ()  [unwired: 5 in, 1 out]
                          }
                          frame #4 {
                            n460 = call "3D_to_Pixels.vi"("X_3D"=0.8 ("element"), "Y_3D"=-0.8 ("element"), "Z_3D"=-0.8 ("element")) -> ("X_pixels"=w1246:dbl, "Y_pixels"=w1245:dbl, "Z_pixels"=w1244:dbl)  [unwired: 9 in, 1 out]
                            n461 = Build Array(w1246, w1245, w1244) -> (w1240:dbl[])
                            n462 = call-poly <vilib>:"Write To Spreadsheet File.vi"("append to file? (new file:F)"=TRUE, "1D data"=w1240, "file path (dialog if empty)"=w1247) -> ()  [unwired: 5 in, 1 out]
                          }
                        }
                      }
                    }
                  }
                }
              }
              frame 6 {
                n463 = Unbundle(w1256) -> ("X_3D"=w1272:dbl, "Y_3D"=w1271:dbl, "Z_3D"=w1270:dbl)
                n464 = call "3D_Session_Data.vi"("Session"=w1257) -> ("Radius"=w1255:sgl, "min"=w1262:dbl, "max"=w1261:dbl)  [unwired: 8 in]
                n465 = Less Or Equal?(x=w1271, y=w1261) -> (x <= y?=w1266:bool)
                n466 = Greater Or Equal?(x=w1271, y=w1262) -> (x >= y?=w1267:bool)
                n467 = Negate(x=w1261) -> (-x=w1260:dbl)
                n468 = Negate(x=w1262) -> (-x=w1259:dbl)
                n469 = Greater Or Equal?(x=w1272, y=w1260) -> (x >= y?=w1269:bool)
                n470 = Less Or Equal?(x=w1272, y=w1259) -> (x <= y?=w1268:bool)
                n471 = Greater Or Equal?(x=w1270, y=w1260) -> (x >= y?=w1265:bool)
                n472 = Less Or Equal?(x=w1270, y=w1259) -> (x <= y?=w1264:bool)
                n473 = Build Array(w1269, w1268, w1267, w1266, w1265, w1264) -> (w1263:bool[])
                n474 = And Array Elements(Boolean array=w1263) -> (logical AND=w1258:bool)
                n475 = case shown="True" w1258 {
                  tunnel: [T12[] [{"Red"=0.0, "Green"=0.0, "Blue"=0.545, "Alpha"=0.8}, {"Red"=0.0, "Green"=0.0, "Blue"=0.545, "Alpha"=0.8}, {"Red"=0.0, "Green"=0.0, "Blue"=0.545, "Alpha"=0.8}, {"Red"=0.0, "Green"=0.0, "Blue"=0.545, "Alpha"=0.8}, {"Red"=0.0, "Green"=0.0, "Blue"=0.545, "Alpha"=0.8}, {"Red"=0.0, "Green"=0.0, "Blue"=0.545, "Alpha"=0.8}, {"Red"=0.0, "Green"=1.0, "Blue"=1.0, "Alpha"=0.8}, {"Red"=0.0, "Green"=0.0, "Blue"=0.545, "Alpha"=0.8}] ("Array") w1334] -> w1289
                  tunnel: [T11 {"Red"=1.0, "Green"=0.0, "Blue"=0.0, "Alpha"=1.0} ("Color") w1333] -> w1288
                  tunnel: w1287 -> [w1297 w1332]
                  tunnel: w1286 -> [w1302 w1331]
                  tunnel: [w1302 w1330] -> w1285
                  tunnel: w1284 -> [w1301 w1329]
                  tunnel: [w1301 w1328] -> w1283
                  tunnel: w1282 -> [_ w1327]
                  tunnel: w1255 -> [_ w1326]
                  tunnel: [w1300 w1325] -> w1281
                  tunnel: w1280 -> [w1300 w1324]
                  tunnel: w1279 -> [w1296 w1323]
                  tunnel: w1278 -> [w1295 w1322]
                  tunnel: [w1294 w1323] -> w1277
                  tunnel: [w1293 w1321] -> w1276
                  tunnel: w1256 -> [w1292 w1320]
                  tunnel: [w1292 w1319] -> w1275
                  tunnel: w1274 -> [w1291 w1318]
                  tunnel: [w1291 w1317] -> w1273
                  frame False {
                    n476 = case shown="False" w1297 {
                      tunnel: w1296 -> [w1305 w1316]
                      tunnel: [w1304 w1315] -> w1294
                      tunnel: w1295 -> [w1307 w1314]
                      tunnel: [w1306 w1314] -> w1293
                      frame False {
                        n477 = Greater Than 0?(x=w1305) -> (x > 0?=w1308:bool)
                        n478 = case shown="True" w1308 {
                          tunnel: w1307 -> [w1310 w1313]
                          tunnel: [w1310 w1312] -> w1306
                          tunnel: w1305 -> [w1309 _]
                          tunnel: [w1309 0 ("y")] -> w1304
                          frame False {
                          }
                          frame True {
                            n479 = Increment(x=w1313) -> (x+1=w1312:i32)
                          }
                        }
                      }
                      frame True {
                        n480 = Increment(x=w1316) -> (x+1=w1315:i32)
                      }
                    }
                    n481 = Number To Decimal String(number=0) -> (decimal integer string=w1299:string)  [unwired: 1 in]
                    n482 = property on="initial time 2" class="DigNum (strict)"("NumText.Text"=w1299) -> ()  [unwired: 2 in, 2 out]
                  }
                  frame True {
                    n483 = case shown="True" w1332 {
                      tunnel: [T12[] [{"Red"=0.0, "Green"=0.0, "Blue"=0.545, "Alpha"=0.8}, {"Red"=0.0, "Green"=0.0, "Blue"=0.545, "Alpha"=0.8}, {"Red"=0.0, "Green"=0.0, "Blue"=0.545, "Alpha"=0.8}, {"Red"=0.0, "Green"=0.0, "Blue"=0.545, "Alpha"=0.8}, {"Red"=0.0, "Green"=0.0, "Blue"=0.545, "Alpha"=0.8}, {"Red"=0.0, "Green"=0.0, "Blue"=0.545, "Alpha"=0.8}, {"Red"=0.0, "Green"=0.8, "Blue"=0.0, "Alpha"=0.8}, {"Red"=0.0, "Green"=0.0, "Blue"=0.545, "Alpha"=0.8}] ("Array") T12[] [{"Red"=0.0, "Green"=0.0, "Blue"=0.545, "Alpha"=0.8}, {"Red"=0.0, "Green"=0.0, "Blue"=0.545, "Alpha"=0.8}, {"Red"=0.0, "Green"=0.0, "Blue"=0.545, "Alpha"=0.8}, {"Red"=0.0, "Green"=0.0, "Blue"=0.545, "Alpha"=0.8}, {"Red"=0.0, "Green"=0.0, "Blue"=0.545, "Alpha"=0.8}, {"Red"=0.0, "Green"=0.0, "Blue"=0.545, "Alpha"=0.8}, {"Red"=1.0, "Green"=1.0, "Blue"=0.0, "Alpha"=0.8}, {"Red"=0.0, "Green"=0.0, "Blue"=0.545, "Alpha"=0.8}] ("Array")] -> w1334
                      tunnel: [T11 {"Red"=0.0, "Green"=0.8, "Blue"=0.0, "Alpha"=1.0} ("Color") T11 {"Red"=1.0, "Green"=1.0, "Blue"=0.0, "Alpha"=1.0} ("Color")] -> w1333
                      tunnel: w1331 -> [w1345 w1370]
                      tunnel: [w1345 w1369] -> w1330
                      tunnel: w1329 -> [w1344 w1368]
                      tunnel: [w1344 w1367] -> w1328
                      tunnel: w1327 -> [_ w1361]
                      tunnel: w1326 -> [_ w1360]
                      tunnel: [w1340 w1359] -> w1325
                      tunnel: w1324 -> [w1339 w1358]
                      tunnel: w1322 -> [w1338 w1357]
                      tunnel: [w1338 0 ("y")] -> w1321
                      tunnel: w1320 -> [w1337 _]
                      tunnel: [w1337 cluster{dbl, dbl, "y":dbl} {0.8, 0.8, "y"=-0.8}] -> w1319
                      tunnel: w1318 -> [w1336 w1354]
                      tunnel: [w1336 w1353] -> w1317
                      frame False {
                        n484 = property on="initial time 2" class="DigNum (strict)"() -> ("NumText.Text"=w1342:string)  [unwired: 2 in, 2 out]
                        n485 = Decimal String To Number(string=w1342) -> (number=w1341:i32)  [unwired: 2 in, 1 out]
                        n486 = Equal To 0?(x=w1341) -> (x = 0?=w1343:bool)
                        n487 = case shown="False" w1343 {
                          tunnel: w1339 -> [w1347 w1351]
                          tunnel: [w1347 w1350] -> w1340
                          frame False {
                          }
                          frame True {
                            n488 = Increment(x=w1351) -> (x+1=w1350:u32)
                            n489 = Number To Decimal String(number=1) -> (decimal integer string=w1349:string)  [unwired: 1 in]
                            n490 = property on="initial time 2" class="DigNum (strict)"("NumText.Text"=w1349) -> ()  [unwired: 2 in, 2 out]
                          }
                        }
                      }
                      frame True {
                        n491 = stacked-sequence {
                          seq-local: [w1417 _] -> [_ w1420]
                          tunnel: [w1416 _] -> w1362
                          frame #0 {
                            n492 = property on="initial time" class="DigNum (strict)"() -> ("NumText.Text"=w1419:string)  [unwired: 2 in, 2 out]
                            n493 = Decimal String To Number(string=w1419) -> (number=w1418:i32)  [unwired: 2 in, 1 out]
                            n494 = Tick Count (ms)() -> (millisecond timer value=w1417:u32)
                            n495 = Subtract(x=w1417, y=w1418) -> (x-y=w1416:u32)
                          }
                          frame #1 {
                            n496 = Number To Decimal String(number=w1420) -> (decimal integer string=w1421:string)  [unwired: 1 in]
                            n497 = property on="initial time" class="DigNum (strict)"("NumText.Text"=w1421) -> ()  [unwired: 2 in, 2 out]
                          }
                        }
                        n498 = Increment(x=w1368) -> (x+1=w1367:i32)
                        n499 = Increment(x=w1370) -> (x+1=w1369:i32)
                        n500 = Current VI's Path() -> (path=w1365:path)
                        n501 = Strip Path(path=w1365) -> (stripped path=w1364:path)  [unwired: 1 out]
                        n502 = Build Path(base path=w1364, name or relative path="successful_hit.wav") -> (appended path=w1366:path)
                        n503 = call <vilib>:"Play Sound File.vi"("path"=w1366) -> ()  [unwired: 9 in, 2 out]
                        n504 = stacked-sequence {
                          tunnel: w1361 -> [w1373 w1384 w1395 w1405 w1414]
                          tunnel: w1362 -> [_ w1382 _ _ _]
                          tunnel: w1360 -> [_ _ w1392 _ _]
                          tunnel: [_ _ w1393 _ _] -> w1359
                          tunnel: w1358 -> [_ _ w1394 _ _]
                          tunnel: w1357 -> [_ w1377 _ _ _]
                          tunnel: w1354 -> [w1374 _ _ _ _]
                          tunnel: [dbl[][] [] _ _ _ _] -> w1353
                          frame #0 {
                            n505 = call-poly <vilib>:"Write To Spreadsheet File.vi"("append to file? (new file:F)"=TRUE, "2D data"=w1374, "file path (dialog if empty)"=w1373) -> ()  [unwired: 5 in, 1 out]
                          }
                          frame #1 {
                            n506 = Greater?(x=w1377, y=u32 10000 ("element")) -> (0:w1380:bool)
                            n507 = Select(t=1, s=w1380, f=w1377) -> (s? t:f=w1376:i32)
                            n508 = Build Array(w1382, w1376, u32 0 ("element")) -> (w1383:u32[])
                            n509 = call-poly <vilib>:"Write To Spreadsheet File.vi"("append to file? (new file:F)"=TRUE, "1D data"=w1383, "file path (dialog if empty)"=w1384) -> ()  [unwired: 5 in, 1 out]
                          }
                          frame #2 {
                            w1393 = u32 0 ("element")
                            n510 = call "3D_to_Pixels.vi"("Distance_3D"=w1392) -> ("Distance_pixels"=w1391:dbl)  [unwired: 11 in, 3 out]
                            n511 = Decrement(x=w1394) -> (x-1=w1387:u32)
                            n512 = Greater?(x=w1387, y=u32 10000 ("element")) -> (0:w1390:bool)
                            n513 = Select(t=1, s=w1390, f=w1387) -> (s? t:f=w1386:u32)
                            n514 = Build Array(w1391, w1386, w1393) -> (w1396:dbl[])
                            n515 = call-poly <vilib>:"Write To Spreadsheet File.vi"("append to file? (new file:F)"=TRUE, "1D data"=w1396, "file path (dialog if empty)"=w1395) -> ()  [unwired: 5 in, 1 out]
                          }
                          frame #3 {
                            n516 = call "3D_to_Pixels.vi"("X_3D"=0.8 ("element"), "Y_3D"=-0.8 ("element"), "Z_3D"=0.8 ("element")) -> ("X_pixels"=w1404:dbl, "Y_pixels"=w1403:dbl, "Z_pixels"=w1402:dbl)  [unwired: 9 in, 1 out]
                            n517 = Build Array(w1404, w1403, w1402) -> (w1398:dbl[])
                            n518 = call-poly <vilib>:"Write To Spreadsheet File.vi"("append to file? (new file:F)"=TRUE, "1D data"=w1398, "file path (dialog if empty)"=w1405) -> ()  [unwired: 5 in, 1 out]
                          }
                          frame #4 {
                            n519 = call "3D_to_Pixels.vi"("X_3D"=-0.8 ("element"), "Y_3D"=0.8 ("element"), "Z_3D"=-0.8 ("element")) -> ("X_pixels"=w1413:dbl, "Y_pixels"=w1412:dbl, "Z_pixels"=w1411:dbl)  [unwired: 9 in, 1 out]
                            n520 = Build Array(w1413, w1412, w1411) -> (w1407:dbl[])
                            n521 = call-poly <vilib>:"Write To Spreadsheet File.vi"("append to file? (new file:F)"=TRUE, "1D data"=w1407, "file path (dialog if empty)"=w1414) -> ()  [unwired: 5 in, 1 out]
                          }
                        }
                      }
                    }
                  }
                }
              }
              frame 7, Default {
                n522 = Unbundle(w1424) -> ("X_3D"=w1439:dbl, "Y_3D"=w1438:dbl, "Z_3D"=w1437:dbl)
                n523 = call "3D_Session_Data.vi"("Session"=w1423) -> ("Radius"=w1422:sgl, "min"=w1427:dbl, "max"=w1426:dbl)  [unwired: 8 in]
                n524 = Less Or Equal?(x=w1437, y=w1426) -> (x <= y?=w1431:bool)
                n525 = Greater Or Equal?(x=w1437, y=w1427) -> (x >= y?=w1432:bool)
                n526 = Negate(x=w1426) -> (-x=w1429:dbl)
                n527 = Negate(x=w1427) -> (-x=w1428:dbl)
                n528 = Greater Or Equal?(x=w1439, y=w1429) -> (x >= y?=w1436:bool)
                n529 = Less Or Equal?(x=w1439, y=w1428) -> (x <= y?=w1435:bool)
                n530 = Greater Or Equal?(x=w1438, y=w1429) -> (x >= y?=w1434:bool)
                n531 = Less Or Equal?(x=w1438, y=w1428) -> (x <= y?=w1433:bool)
                n532 = Build Array(w1436, w1435, w1434, w1433, w1432, w1431) -> (w1430:bool[])
                n533 = And Array Elements(Boolean array=w1430) -> (logical AND=w1425:bool)
                n534 = case shown="False" w1425 {
                  tunnel: [T12[] [{"Red"=0.0, "Green"=0.0, "Blue"=0.545, "Alpha"=0.8}, {"Red"=0.0, "Green"=1.0, "Blue"=1.0, "Alpha"=0.8}, {"Red"=0.0, "Green"=0.0, "Blue"=0.545, "Alpha"=0.8}, {"Red"=0.0, "Green"=0.0, "Blue"=0.545, "Alpha"=0.8}, {"Red"=0.0, "Green"=0.0, "Blue"=0.545, "Alpha"=0.8}, {"Red"=0.0, "Green"=0.0, "Blue"=0.545, "Alpha"=0.8}, {"Red"=0.0, "Green"=0.0, "Blue"=0.545, "Alpha"=0.8}, {"Red"=0.0, "Green"=0.0, "Blue"=0.545, "Alpha"=0.8}] ("Array") w1501] -> w1456
                  tunnel: [T11 {"Red"=1.0, "Green"=0.0, "Blue"=0.0, "Alpha"=1.0} ("Color") w1500] -> w1455
                  tunnel: w1454 -> [w1464 w1499]
                  tunnel: w1453 -> [w1469 w1498]
                  tunnel: [w1469 w1497] -> w1452
                  tunnel: w1451 -> [w1468 w1496]
                  tunnel: [w1468 w1495] -> w1450
                  tunnel: w1449 -> [_ w1494]
                  tunnel: w1422 -> [_ w1493]
                  tunnel: w1448 -> [w1467 w1492]
                  tunnel: [w1467 w1491] -> w1447
                  tunnel: w1446 -> [w1463 w1490]
                  tunnel: w1445 -> [w1462 w1489]
                  tunnel: [w1461 w1488] -> w1444
                  tunnel: [w1460 w1490] -> w1443
                  tunnel: w1424 -> [w1459 w1487]
                  tunnel: [w1459 w1486] -> w1442
                  tunnel: w1441 -> [w1458 w1485]
                  tunnel: [w1458 w1484] -> w1440
                  frame False {
                    n535 = case shown="False" w1464 {
                      tunnel: w1463 -> [w1472 w1483]
                      tunnel: [w1471 w1482] -> w1460
                      tunnel: w1462 -> [w1474 w1481]
                      tunnel: [w1473 w1481] -> w1461
                      frame False {
                        n536 = Greater Than 0?(x=w1472) -> (x > 0?=w1475:bool)
                        n537 = case shown="True" w1475 {
                          tunnel: w1474 -> [w1477 w1480]
                          tunnel: [w1477 w1479] -> w1473
                          tunnel: w1472 -> [w1476 _]
                          tunnel: [w1476 0 ("y")] -> w1471
                          frame False {
                          }
                          frame True {
                            n538 = Increment(x=w1480) -> (x+1=w1479:i32)
                          }
                        }
                      }
                      frame True {
                        n539 = Increment(x=w1483) -> (x+1=w1482:i32)
                      }
                    }
                    n540 = Number To Decimal String(number=0) -> (decimal integer string=w1466:string)  [unwired: 1 in]
                    n541 = property on="initial time 2" class="DigNum (strict)"("NumText.Text"=w1466) -> ()  [unwired: 2 in, 2 out]
                  }
                  frame True {
                    n542 = case shown="True" w1499 {
                      tunnel: [T12[] [{"Red"=0.0, "Green"=0.0, "Blue"=0.545, "Alpha"=0.8}, {"Red"=0.0, "Green"=0.8, "Blue"=0.0, "Alpha"=0.8}, {"Red"=0.0, "Green"=0.0, "Blue"=0.545, "Alpha"=0.8}, {"Red"=0.0, "Green"=0.0, "Blue"=0.545, "Alpha"=0.8}, {"Red"=0.0, "Green"=0.0, "Blue"=0.545, "Alpha"=0.8}, {"Red"=0.0, "Green"=0.0, "Blue"=0.545, "Alpha"=0.8}, {"Red"=0.0, "Green"=0.0, "Blue"=0.545, "Alpha"=0.8}, {"Red"=0.0, "Green"=0.0, "Blue"=0.545, "Alpha"=0.8}] ("Array") T12[] [{"Red"=0.0, "Green"=0.0, "Blue"=0.545, "Alpha"=0.8}, {"Red"=1.0, "Green"=1.0, "Blue"=0.0, "Alpha"=0.8}, {"Red"=0.0, "Green"=0.0, "Blue"=0.545, "Alpha"=0.8}, {"Red"=0.0, "Green"=0.0, "Blue"=0.545, "Alpha"=0.8}, {"Red"=0.0, "Green"=0.0, "Blue"=0.545, "Alpha"=0.8}, {"Red"=0.0, "Green"=0.0, "Blue"=0.545, "Alpha"=0.8}, {"Red"=0.0, "Green"=0.0, "Blue"=0.545, "Alpha"=0.8}, {"Red"=0.0, "Green"=0.0, "Blue"=0.545, "Alpha"=0.8}] ("Array")] -> w1501
                      tunnel: [T11 {"Red"=0.0, "Green"=0.8, "Blue"=0.0, "Alpha"=1.0} ("Color") T11 {"Red"=1.0, "Green"=1.0, "Blue"=0.0, "Alpha"=1.0} ("Color")] -> w1500
                      tunnel: w1498 -> [w1512 w1537]
                      tunnel: [w1512 w1536] -> w1497
                      tunnel: w1496 -> [w1511 w1535]
                      tunnel: [w1511 w1534] -> w1495
                      tunnel: w1494 -> [_ w1528]
                      tunnel: w1493 -> [_ w1527]
                      tunnel: w1492 -> [w1506 w1526]
                      tunnel: [w1507 w1525] -> w1491
                      tunnel: w1489 -> [w1505 w1524]
                      tunnel: [w1505 0 ("x")] -> w1488
                      tunnel: w1487 -> [w1504 _]
                      tunnel: [w1504 cluster{dbl, dbl, "y":dbl} {-0.8, -0.8, "y"=0.8}] -> w1486
                      tunnel: w1485 -> [w1503 w1521]
                      tunnel: [w1503 w1520] -> w1484
                      frame False {
                        n543 = property on="initial time 2" class="DigNum (strict)"() -> ("NumText.Text"=w1509:string)  [unwired: 2 in, 2 out]
                        n544 = Decimal String To Number(string=w1509) -> (number=w1508:i32)  [unwired: 2 in, 1 out]
                        n545 = Equal To 0?(x=w1508) -> (x = 0?=w1510:bool)
                        n546 = case shown="False" w1510 {
                          tunnel: w1506 -> [w1514 w1518]
                          tunnel: [w1514 w1517] -> w1507
                          frame False {
                          }
                          frame True {
                            n547 = Increment(x=w1518) -> (x+1=w1517:u32)
                            n548 = Number To Decimal String(number=1) -> (decimal integer string=w1516:string)  [unwired: 1 in]
                            n549 = property on="initial time 2" class="DigNum (strict)"("NumText.Text"=w1516) -> ()  [unwired: 2 in, 2 out]
                          }
                        }
                      }
                      frame True {
                        n550 = stacked-sequence {
                          seq-local: [w1584 _] -> [_ w1587]
                          tunnel: [w1583 _] -> w1529
                          frame #0 {
                            n551 = property on="initial time" class="DigNum (strict)"() -> ("NumText.Text"=w1586:string)  [unwired: 2 in, 2 out]
                            n552 = Decimal String To Number(string=w1586) -> (number=w1585:i32)  [unwired: 2 in, 1 out]
                            n553 = Tick Count (ms)() -> (millisecond timer value=w1584:u32)
                            n554 = Subtract(x=w1584, y=w1585) -> (x-y=w1583:u32)
                          }
                          frame #1 {
                            n555 = Number To Decimal String(number=w1587) -> (decimal integer string=w1588:string)  [unwired: 1 in]
                            n556 = property on="initial time" class="DigNum (strict)"("NumText.Text"=w1588) -> ()  [unwired: 2 in, 2 out]
                          }
                        }
                        n557 = Increment(x=w1535) -> (x+1=w1534:i32)
                        n558 = Increment(x=w1537) -> (x+1=w1536:i32)
                        n559 = Current VI's Path() -> (path=w1532:path)
                        n560 = Strip Path(path=w1532) -> (stripped path=w1531:path)  [unwired: 1 out]
                        n561 = Build Path(base path=w1531, name or relative path="successful_hit.wav") -> (appended path=w1533:path)
                        n562 = call <vilib>:"Play Sound File.vi"("path"=w1533) -> ()  [unwired: 9 in, 2 out]
                        n563 = stacked-sequence {
                          tunnel: w1528 -> [w1541 w1551 w1562 w1572 w1581]
                          tunnel: w1529 -> [_ w1549 _ _ _]
                          tunnel: w1527 -> [_ _ w1559 _ _]
                          tunnel: w1526 -> [_ _ w1561 _ _]
                          tunnel: [_ _ w1560 _ _] -> w1525
                          tunnel: w1524 -> [_ w1544 _ _ _]
                          tunnel: w1521 -> [w1540 _ _ _ _]
                          tunnel: [dbl[][] [] _ _ _ _] -> w1520
                          frame #0 {
                            n564 = call-poly <vilib>:"Write To Spreadsheet File.vi"("append to file? (new file:F)"=TRUE, "2D data"=w1540, "file path (dialog if empty)"=w1541) -> ()  [unwired: 5 in, 1 out]
                          }
                          frame #1 {
                            n565 = Greater?(x=w1544, y=u32 10000 ("element")) -> (0:w1547:bool)
                            n566 = Select(t=1, s=w1547, f=w1544) -> (s? t:f=w1543:i32)
                            n567 = Build Array(w1549, w1543, u32 0 ("element")) -> (w1550:u32[])
                            n568 = call-poly <vilib>:"Write To Spreadsheet File.vi"("append to file? (new file:F)"=TRUE, "1D data"=w1550, "file path (dialog if empty)"=w1551) -> ()  [unwired: 5 in, 1 out]
                          }
                          frame #2 {
                            w1560 = u32 0 ("element")
                            n569 = call "3D_to_Pixels.vi"("Distance_3D"=w1559) -> ("Distance_pixels"=w1558:dbl)  [unwired: 11 in, 3 out]
                            n570 = Decrement(x=w1561) -> (x-1=w1554:u32)
                            n571 = Greater?(x=w1554, y=u32 10000 ("element")) -> (0:w1557:bool)
                            n572 = Select(t=1, s=w1557, f=w1554) -> (s? t:f=w1553:u32)
                            n573 = Build Array(w1558, w1553, w1560) -> (w1563:dbl[])
                            n574 = call-poly <vilib>:"Write To Spreadsheet File.vi"("append to file? (new file:F)"=TRUE, "1D data"=w1563, "file path (dialog if empty)"=w1562) -> ()  [unwired: 5 in, 1 out]
                          }
                          frame #3 {
                            n575 = call "3D_to_Pixels.vi"("X_3D"=0.8 ("element"), "Y_3D"=0.8 ("element"), "Z_3D"=-0.8 ("element")) -> ("X_pixels"=w1571:dbl, "Y_pixels"=w1570:dbl, "Z_pixels"=w1569:dbl)  [unwired: 9 in, 1 out]
                            n576 = Build Array(w1571, w1570, w1569) -> (w1568:dbl[])
                            n577 = call-poly <vilib>:"Write To Spreadsheet File.vi"("append to file? (new file:F)"=TRUE, "1D data"=w1568, "file path (dialog if empty)"=w1572) -> ()  [unwired: 5 in, 1 out]
                          }
                          frame #4 {
                            n578 = call "3D_to_Pixels.vi"("X_3D"=-0.8 ("element"), "Y_3D"=-0.8 ("element"), "Z_3D"=0.8 ("element")) -> ("X_pixels"=w1580:dbl, "Y_pixels"=w1579:dbl, "Z_pixels"=w1578:dbl)  [unwired: 9 in, 1 out]
                            n579 = Build Array(w1580, w1579, w1578) -> (w1577:dbl[])
                            n580 = call-poly <vilib>:"Write To Spreadsheet File.vi"("append to file? (new file:F)"=TRUE, "1D data"=w1577, "file path (dialog if empty)"=w1581) -> ()  [unwired: 5 in, 1 out]
                          }
                        }
                      }
                    }
                  }
                }
              }
            }
          }
        }
        n581 = for {
          tunnel: w176 -> [w194] mode=indexing
          tunnel: w175 -> [w197] mode=indexing
          tunnel: w173 -> [w196]
          tunnel: w172 -> [w195] mode=indexing
          n582 = property class="SceneObject"(reference=w194, "Material.Diffuse"=w197) -> ()  [unwired: 1 in, 2 out]
          n583 = property class="SceneSphere"(reference=w195, "Radius"=w196) -> ()  [unwired: 1 in, 2 out]
        }
        n584 = call <vilib>:"Set Translation.vi"("Translation"=w122, "Scene Object"=w179) -> ("Translated Object"=w177:refnum<vi>)  [unwired: 8 in, 1 out]
        n585 = property class="SceneSphere"(reference=w174, "Radius"=w173) -> ()  [unwired: 1 in, 2 out]
        n586 = property class="SceneObject"(reference=w177, "Material.Diffuse"=w178) -> ()  [unwired: 1 in, 2 out]
        n587 = node-c288() -> ()  [unwired: 1 in, 1 out]
        "3D Picture" <- w180
      }
      n588 = node-c288(w106) -> ()  [unwired: 1 out]
    }
    frame #2 {
      n589 = call "Time Delay2"() -> ()  [unwired: 11 in, 1 out]
    }
  }
  n590 = property class="VI"(reference=w4, error in=w3, "Front Panel Window:Open"=TRUE) -> (reference out=w7:refnum<vi>, error out=w6:errorcluster)
  n591 = Close Reference(reference=w7, error in (no error)=w6) -> ()  [unwired: 1 out]
